vi "svx_Polar_Property_Dialog.vi"(0 "Data in":T1, 1 "Container State in":T2 caption="Container State", 2 "Polar Plot":refnum<vi>, 3 "Plot Legend":refnum<vi>, 4 "z scale graph ref in":refnum<vi>, 5 "This VI":refnum<vi>, 6 "State in":T4={"Property Name"=[], "Container bounds"={"Width"=550, "Height"=250}, "Scale range"={"Maximum"=1.0, "Increment"=1.0}, "PointIdx"=0, "Marker list"=[], "Color settings"={"Arrow color"=16860, "Magnitude major grid"=13816530, "Magnitude minor grid"=16777216, "Phase grid"=13816530, "Phase scale marker text"=0}, "Magnitude scale name"="Magnitude", "Magnitude scale format string"="%#.2e", "MagnitudeScale:Visible"=TRUE, "MagnitudeScaleLabel:Visible"=TRUE, "PhaseScale:Visible"=TRUE, "Marker:Visible"=TRUE, "Cursor:Visible"=FALSE, "CursorName:Visible"=TRUE, "Autoscale"=TRUE, "Marker color"=16860, "Line color"=16711680, "Cursor color"=16711680, "Magnitude scale marker color"=0, "Plot.Line Style"=0, "Plot.Line Width"=0, "Plot.Point Style"=0, "Cursor.Line Style"=0, "Cursor.Line Width"=0, "Cursor.Point Style"=0, "Cursor.Style"=4, "Marker.Point Style"=2, "Point/fill color"=16711680, "Background color"=16777225, "Cursor name"="", "Cursor Release"=refnum, "Scale Range Change"=refnum, "data size(s)"=[], "Selectors:Visible"=TRUE, "Selector:ring Strings"={"Selector:Custom Strings"=FALSE, "Selector:Row Strings []"=[], "Selector:Column Strings []"=[], "User:Row Strings []"=[], "User:Column Strings []"=[]}, "Lock Cursor Info Position"=FALSE, "CursLoc"={"magnitude"=0.0, "phase"=0.0, "time/rev/RPM"=0.0}, "Plot Area:Position"={"Left"=0, "Top"=0}, "Plot Area:Size"={"Width"=0, "Height"=0}, "Marker.Style"=0, "Indication Arcs"=[], "Arc.Selector"=0, "customized marker"=[], "tree Width"=0, " Parents Tags"=[], "Children Tags"=[], "open?"=[], "index"=[{"row index"=0, "column index"=0}], "Label"="", "custom strings changed"=FALSE, "Owning VI"=refnum, "Legend BG color"=16777225, "Legend font color"=0, "column Width"=203, "attribute"=variant} caption="State", 7 "Action in":T3, 8 "acceptance region only?":bool, 9 "Cursor Info":refnum<vi>) -> (12 "State out":T4={"Property Name"=[], "Container bounds"={"Width"=550, "Height"=250}, "Scale range"={"Maximum"=1.0, "Increment"=1.0}, "PointIdx"=0, "Marker list"=[], "Color settings"={"Arrow color"=16860, "Magnitude major grid"=13816530, "Magnitude minor grid"=16777216, "Phase grid"=13816530, "Phase scale marker text"=0}, "Magnitude scale name"="Magnitude", "Magnitude scale format string"="%#.2e", "MagnitudeScale:Visible"=TRUE, "MagnitudeScaleLabel:Visible"=TRUE, "PhaseScale:Visible"=TRUE, "Marker:Visible"=TRUE, "Cursor:Visible"=FALSE, "CursorName:Visible"=TRUE, "Autoscale"=TRUE, "Marker color"=16860, "Line color"=16711680, "Cursor color"=16711680, "Magnitude scale marker color"=0, "Plot.Line Style"=0, "Plot.Line Width"=0, "Plot.Point Style"=0, "Cursor.Line Style"=0, "Cursor.Line Width"=0, "Cursor.Point Style"=0, "Cursor.Style"=4, "Marker.Point Style"=2, "Point/fill color"=16711680, "Background color"=16777225, "Cursor name"="", "Cursor Release"=refnum, "Scale Range Change"=refnum, "data size(s)"=[], "Selectors:Visible"=TRUE, "Selector:ring Strings"={"Selector:Custom Strings"=FALSE, "Selector:Row Strings []"=[], "Selector:Column Strings []"=[], "User:Row Strings []"=[], "User:Column Strings []"=[]}, "Lock Cursor Info Position"=FALSE, "CursLoc"={"magnitude"=0.0, "phase"=0.0, "time/rev/RPM"=0.0}, "Plot Area:Position"={"Left"=0, "Top"=0}, "Plot Area:Size"={"Width"=0, "Height"=0}, "Marker.Style"=0, "Indication Arcs"=[], "Arc.Selector"=0, "customized marker"=[], "tree Width"=0, " Parents Tags"=[], "Children Tags"=[], "open?"=[], "index"=[{"row index"=0, "column index"=0}], "Label"="", "custom strings changed"=FALSE, "Owning VI"=refnum, "Legend BG color"=16777225, "Legend font color"=0, "column Width"=203, "attribute"=variant} caption="State", 13 "Action out":T3, 14 "Data out":T1)   [LabVIEW 2017, in "SVX Polar Plot.xctl"]
uses:
  <vilib>/addons/_XControls/Polar Plot/SVX Polar Plot.xctl
  <vilib>/addons/_XControls/Polar Plot/subVIs/svx_Polar_Plot_Internal_State.ctl
  <vilib>/addons/_XControls/Polar Plot/subVIs/svx_Polar_Indication_Arcs.ctl
  <vilib>/addons/_XControls/Polar Plot/subVIs/svx_Polar_Customized_Markers.ctl
  <vilib>/_xctls/Action.ctl
  <vilib>/_xctls/Container State.ctl
  <vilib>/addons/_XControls/Polar Plot/subVIs/svx_Polar_Plot_Data.ctl
  <vilib>/addons/_XControls/Polar Plot/subVIs/svx_Polar_Exe_Tasks.ctl
  <vilib>/_xctls/XControlSupport.lvlib
panel:
  out "update maximum value":bool
  in  "Help":bool
  in  "Cancel":bool
  in  "OK":bool
  in  "Main Tab":T7(tab)
  in  "Plot Legend Font.Color":u32(colorbox)=16777222 caption="Legend font"
  in  "Plot Legend Background.Color":u32(colorbox)=16777225 caption="Legend background"
  in  "Background.Color":u32(colorbox)=16777225 caption="Background"
  in  "Enable State":T8(radio)
  in  "Arrow.Color":u32(colorbox)=16860 caption="Arrow color"
  in  "Label.Visible":bool=TRUE
  in  "Label.Text":string="Polar Plot"
  in  "Caption.Visible":bool
  in  "Caption.Text":string="Polar Plot"
  in  "Hide trailing zeros":bool=TRUE
  in  "Digits":u8=2
  in  "Precision Type":u16(ring) items=["Digits of precision", "Significant digits"]
  in  "Type":i32(listbox)=2
  in  "Point/Fill.Color":u32(colorbox)=16860 caption="Point/Fill"
  in  "Marker.Point Style":T9 caption="Point Style"
  in  "Line.Color":u32(colorbox)=16860 caption="Line color"
  in  "Plot.Point Style":T9 caption="Point Style"
  in  "Plot.Line Style":T10 caption="Line Style"
  in  "Plot.Line Width":T11 caption="Line Width"
  in  "Marker.Color":u32(colorbox)=16711680 caption="Marker color"
  in  "Marker.Visible":bool=TRUE caption="Show scale label"
  in  "Marker.Style":T12 caption="Cursor Style"
  in  "Magnitude Minor Grid.Color":u32(colorbox)=16777216 caption="Magnitude minor grid"
  in  "Phase Scale.Visible":bool=TRUE caption="Show scale"
  in  "Magnitude Scale Marker Text.Color":u32(colorbox) caption="Magnitude scale marker text"
  in  "Phase Grid.Color":u32(colorbox)=13816530 caption="Phase grid"
  in  "Magnitude Major Grid.Color":u32(colorbox)=13816530 caption="Magnitude major grid"
  in  "Phase Scale Marker Text.Color":u32(colorbox) caption="Phase scale marker text"
  in  "Magnitude Scale Label.Visible":bool=TRUE caption="Show scale label"
  in  "Magnitude Range:Maximum":dbl=10.0 caption="Maximum" min=0.0 format="%0.2f"
  in  "Magnitude.Scale Fit":bool caption="Autoscale"
  in  "Magnitude Scale.Visible":bool=TRUE caption="Show scale"
  in  "Magnitude.Text":string caption="Name"
  in  "Cursor Info Position.Lock":bool caption="Show scale label"
  in  "Cursor.Visible":bool=TRUE caption="Show scale label"
  in  "Cursor.Color":u32(colorbox)=16711680 caption="Cursor color"
  in  "Cursor Info.Visible":bool=TRUE caption="Show scale label"
  in  "Cursor.Style":T12 caption="Cursor Style"
  in  "Cursor.Line Width":T11 caption="Line Width"
  in  "Cursor.Line Style":T10 caption="Line Style"
  in  "Cursor.Point Style":T9 caption="Point Style"
  in  "AR.Selector":u16(ring) caption="Indication Arc" items=["Acceptance Region 0"]
  in  "AR.Fill Color":u32(colorbox)=16777216 caption="Fill color"
  in  "AR.Name":string caption="Name"
  in  "AR.Remove":bool
  in  "AR.Add":bool
  in  "AR.Style":T10 caption="Line Style"
  in  "AR.Width":T11 caption="Line Width"
  in  "AR.Start Radius":dbl caption="Start radius"
  in  "AR.Color":u32(colorbox)=16711680 caption="Border color"
  in  "AR.Start Angle":i16 caption="Start angle" min=-360 max=360
  in  "AR.End Angle":i16=360 caption="End angle" min=-360 max=360
  in  "AR.Visible":bool
  in  "AR.End Radius":dbl caption="End radius"
  in  "Tip strip":string
  in  "Description":string
  # "Label"
  # "Caption"
  # "Enabled State"
  # "Color Scheme"
  # "Magnitude"
  # "Plot"
  # "Color"
  # "Marker"
  # "Magnitude"
  # "Phase"
  # "Cursor"
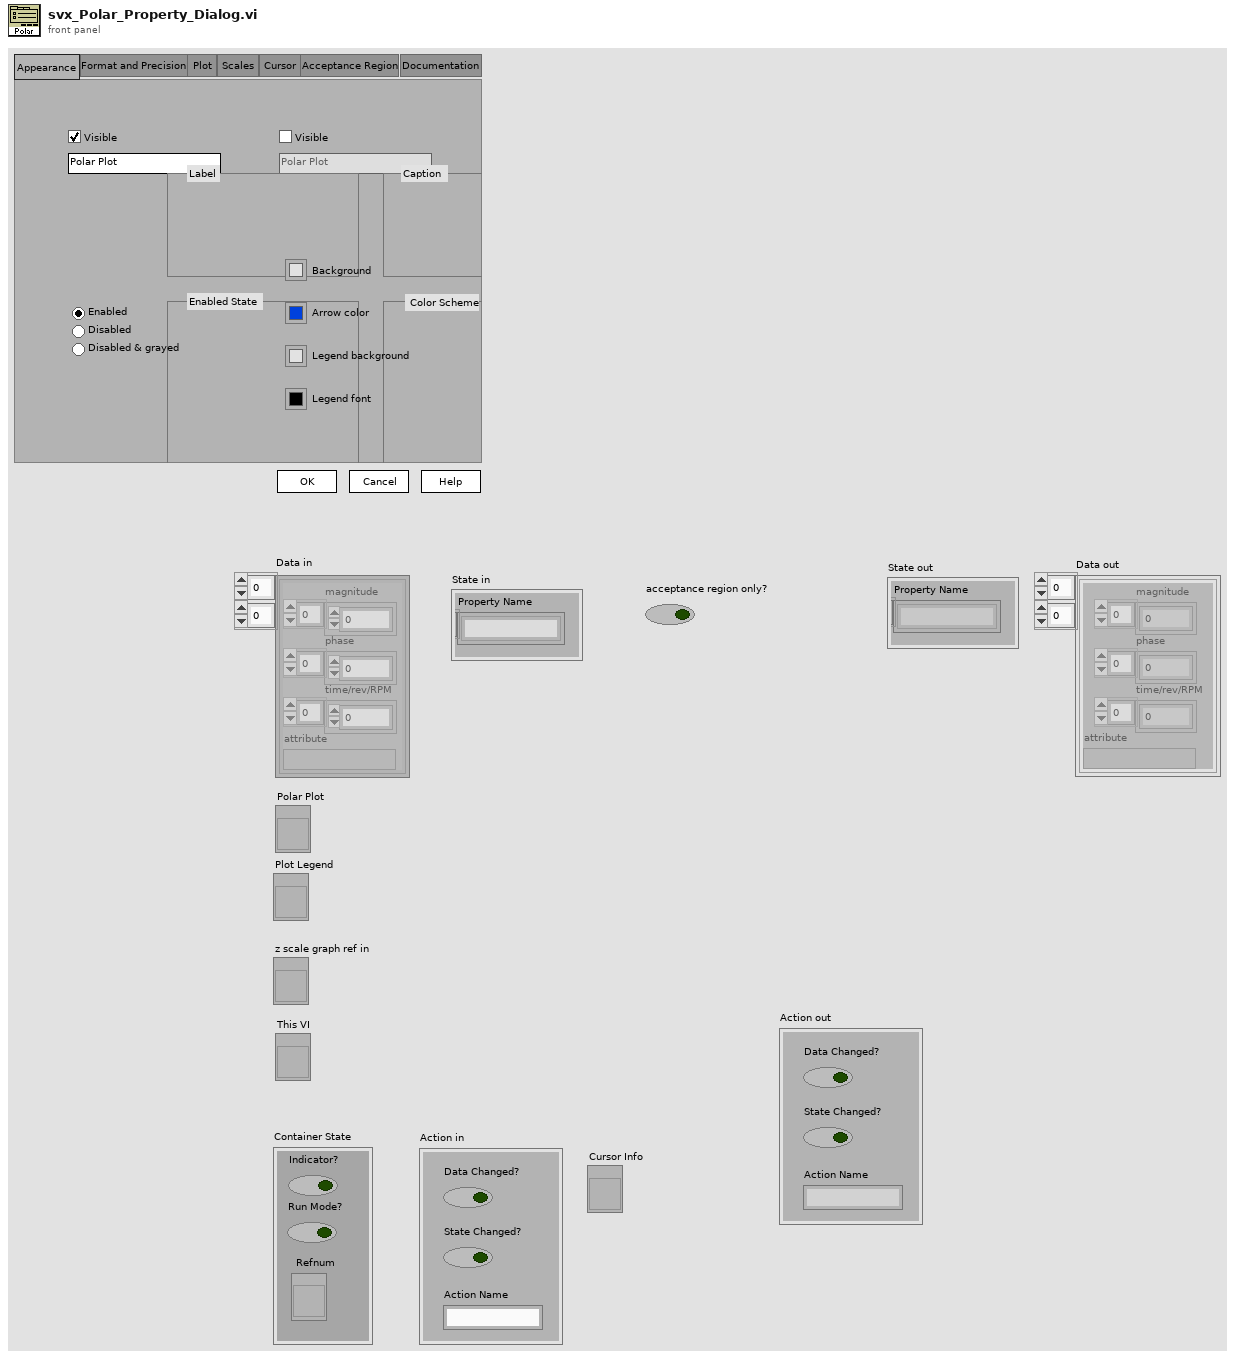
[diagram p1: front panel]
types:
  T1 = typedef "SVX Polar Plot.xctl/svx_Polar_Plot_Data.ctl" = cluster{"magnitude":dbl[], "phase":dbl[], "time/rev/RPM":dbl[], "attribute":variant}[][]
  T2 = typedef "XControlSupport.lvlib/Container State.ctl" = cluster{"Indicator?":bool, "Run Mode?":bool, " Refnum":refnum<vi>}
  T3 = typedef "XControlSupport.lvlib/Action.ctl" = cluster{"Data Changed?":bool, "State Changed?":bool, "Action Name":string}
  T4 = typedef "SVX Polar Plot.xctl/svx_Polar_Plot_Internal_State.ctl" = cluster{"Property Name":string[], "Container bounds":cluster{"Width":u32, "Height":u32}, "Scale range":cluster{"Maximum":dbl, "Increment":dbl}, "PointIdx":i32, "Marker list":cluster{"Name":string, "Color":u32, "Style":u8, "Point Style":u8, "Name Visible":bool, "Allow Drag":bool, "Annotation Mode":u32, "Plot":i32, "Index":i32, "Position":cluster{"X":dbl, "Y":dbl}, "X Scale":u32, "Y Scale":u32, "Show Arrow":bool, "Lock Name":bool, "Plot Area":i32, "Label Offset":cluster{"X":dbl, "Y":dbl}}[], "Color settings":cluster{"Arrow color":u32, "Magnitude major grid":u32, "Magnitude minor grid":u32, "Phase grid":u32, "Phase scale marker text":u32}, "Magnitude scale name":string, "Magnitude scale format string":string, "MagnitudeScale:Visible":bool, "MagnitudeScaleLabel:Visible":bool, "PhaseScale:Visible":bool, "Marker:Visible":bool, "Cursor:Visible":bool, "CursorName:Visible":bool, "Autoscale":bool, "Marker color":u32, "Line color":u32, "Cursor color":u32, "Magnitude scale marker color":u32, "Plot.Line Style":i32, "Plot.Line Width":i32, "Plot.Point Style":i32, "Cursor.Line Style":i32, "Cursor.Line Width":i32, "Cursor.Point Style":i32, "Cursor.Style":i32, "Marker.Point Style":i32, "Point/fill color":u32, "Background color":u32, "Cursor name":string, "Cursor Release":refnum<user-event>, "Scale Range Change":refnum<user-event>, "data size(s)":i32[], "Selectors:Visible":bool, "Selector:ring Strings":cluster{"Selector:Custom Strings":bool, "Selector:Row Strings []":string[], "Selector:Column Strings []":string[], "User:Row Strings []":string[], "User:Column Strings []":string[]}, "Lock Cursor Info Position":bool, "CursLoc":cluster{"magnitude":dbl, "phase":dbl, "time/rev/RPM":dbl}, "Plot Area:Position":cluster{"Left":i32, "Top":i32}, "Plot Area:Size":cluster{"Width":u32, "Height":u32}, "Marker.Style":i32, "Indication Arcs":T5, "Arc.Selector":u16, "customized marker":T6, "tree Width":u32, " Parents Tags":string[], "Children Tags":string[], "open?":bool[], "index":cluster{"row index":i32, "column index":i32}[], "Label":string, "custom strings changed":bool, "Owning VI":refnum<vi>, "Legend BG color":u32, "Legend font color":u32, "column Width":u32, "attribute":variant}
  T5 = typedef "SVX Polar Plot.xctl/svx_Polar_Indication_Arcs.ctl" = cluster{"Name":string, "Start radius":dbl, "End radius":dbl, "Line Style":i32, "Line Width":i32, "Border color":u32, "Fill color":u32, "Start angle":i16, "End angle":i16, "Visible":bool}[]
  T6 = typedef "SVX Polar Plot.xctl/svx_Polar_Customized_Markers.ctl" = cluster{"Name":string, "Color":u32, "Style":u8, "Point Style":u8, "Name Visible":bool, "Allow Drag":bool, "Annotation Mode":u32, "Plot":i32, "Index":i32, "Position":cluster{"Magnitude":dbl, "Phase":dbl}, "X Scale":u32, "Y Scale":u32, "Show Arrow":bool, "Lock Name":bool, "Plot Area":i32, "Label Offset":cluster{"Magnitude":dbl, "Phase":dbl}}[]
  T7 = enum32{"Appearance", "Format and Precision", "Plot", "Scales", "Cursor", "Acceptance Region", "Documentation"}
  T8 = enum32{"Enabled", "Disabled", "Disabled & grayed"}
  T9 = cluster{"OK Button 17":bool, "OK Button":bool, "OK Button 2":bool, "OK Button 3":bool, "OK Button 4":bool, "OK Button 5":bool, "OK Button 6":bool, "OK Button 7":bool, "OK Button 8":bool, "OK Button 9":bool, "OK Button 10":bool, "OK Button 11":bool, "OK Button 12":bool, "OK Button 13":bool, "OK Button 14":bool, "OK Button 15":bool, "OK Button 16":bool}
  T10 = cluster{"OK Button":bool, "OK Button 2":bool, "OK Button 3":bool, "OK Button 4":bool, "OK Button 5":bool}
  T11 = cluster{"OK Button 2":bool, "OK Button 3":bool, "OK Button 4":bool, "OK Button 5":bool, "OK Button 6":bool, "OK Button 7":bool}
  T12 = cluster{"OK Button 17":bool, "OK Button":bool, "OK Button 2":bool, "OK Button 5":bool, "OK Button 13":bool, "OK Button 10":bool, "OK Button 6":bool, "OK Button 9":bool, "OK Button 14":bool}
  T13 = cluster{"Label.Text":string, "Caption.Text":string, "Label.Visible":bool, "Caption.Visible":bool, "Disabled":u8, "Desc":string, "TipStrip":string}
  T14 = cluster{"Name":string, "Start radius":dbl, "End radius":dbl, "Line Style":i32, "Line Width":i32, "Border color":u32, "Fill color":u32, "Start angle":i16, "End angle":i16, "Visible":bool}
  T15 = typedef "SVX Polar Plot.xctl/svx_Polar_Exe_Tasks.ctl" = enum16{"[Data] Update Data", "[Scale] Update Polar Scale", "[Scale] Autoscale", "[Legend] Update Legend", "[Cursor] Cursor Release", "[Pane] Change Minimum Size", "[Annt] Upodate Annotation", "[Plot] Appearance", "[Cursor] Visibility", "[Cursor] Appearance", "[Cursor] Index", "[Scale] MagnitudeVisibility", "[Scale] PhaseVisibility", "[Scale] PhaseAppearance", "[Scale] MagnitudeApperance", "[Plot] AcceptanceRegion", "[Scale] RangeChange", "[Marker] Appearance", "[Marker] List", "[Marker] Visibility", "[Legend] Visibility", "[Legend] Color", "[Data] Index", "[Legend] Update String", "[Cursor] Trigger Event", "[Scale] Trigger Event", "[Data] Clear Graph"}
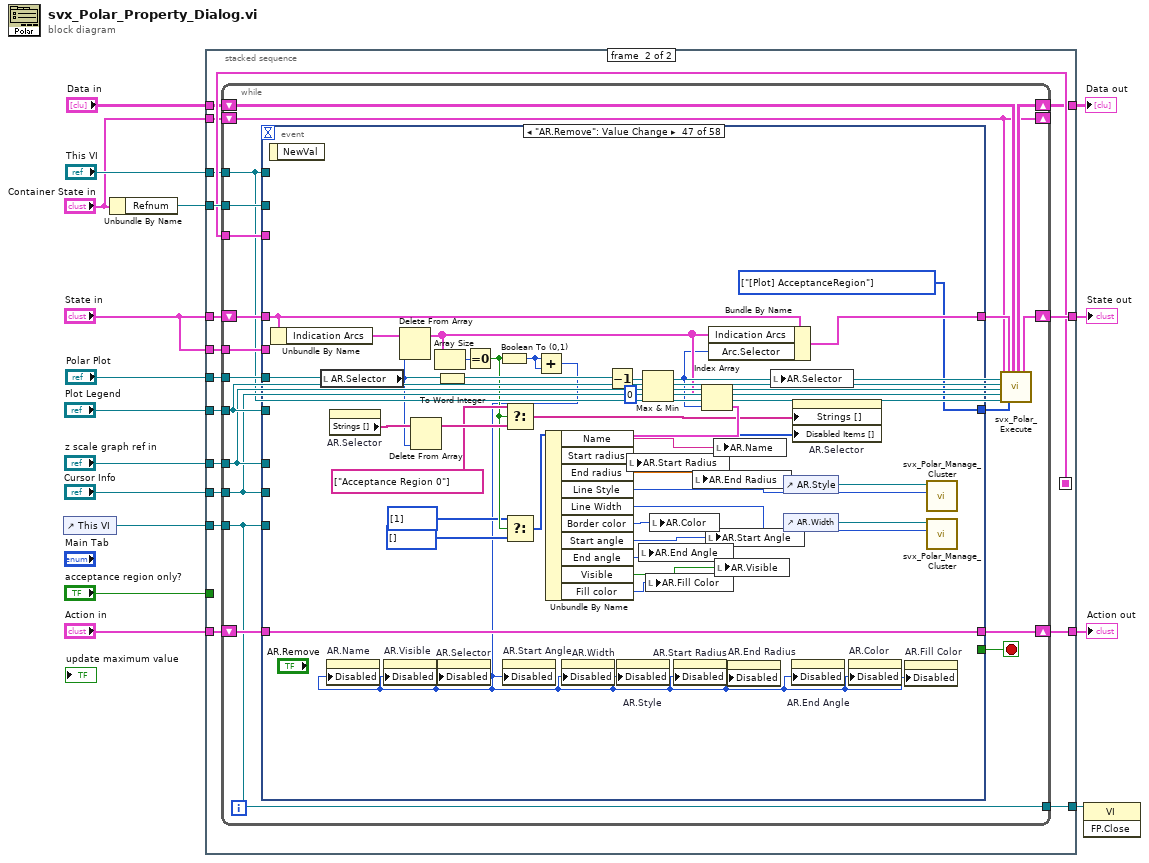
[diagram p0: block diagram]
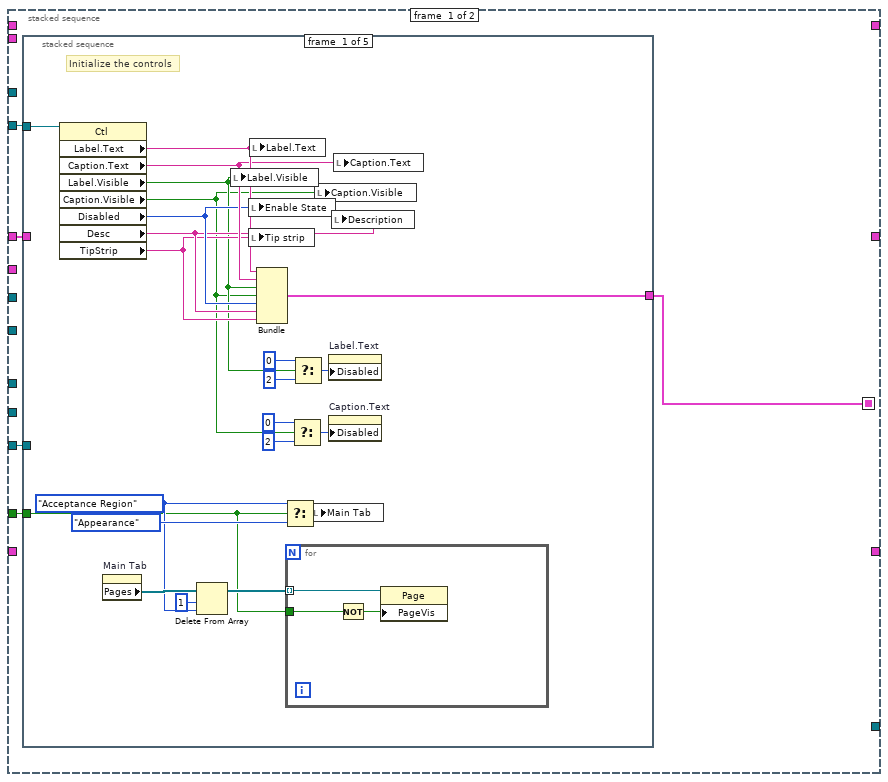
[diagram p2: hidden frame]
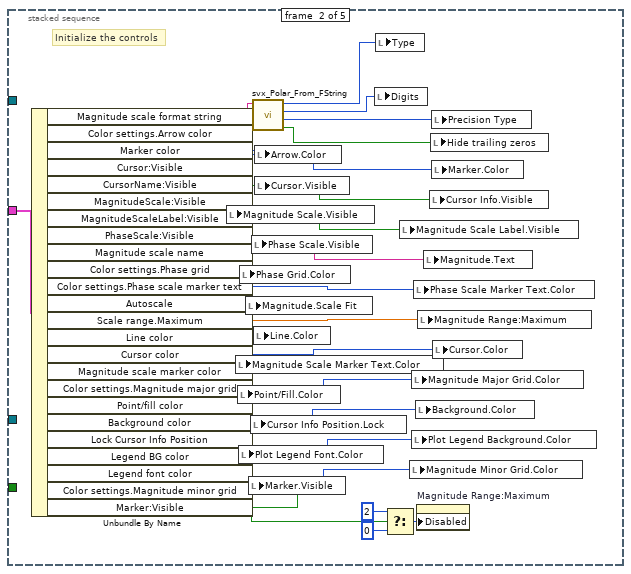
[diagram p3: hidden frame]
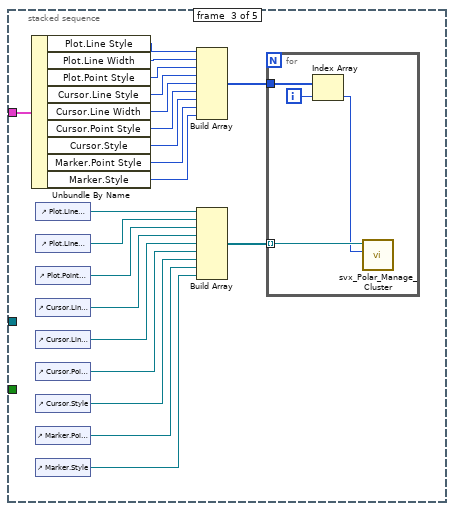
[diagram p4: hidden frame]
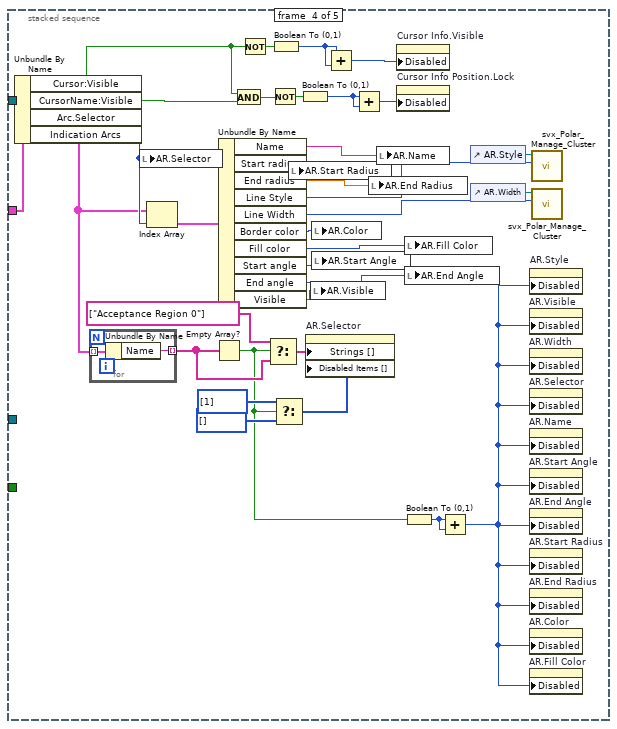
[diagram p5: hidden frame]
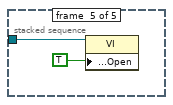
[diagram p6: hidden frame]
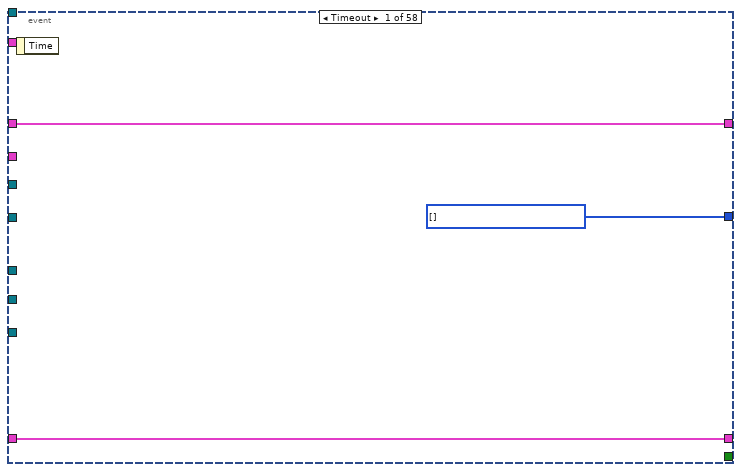
[diagram p7: hidden frame]
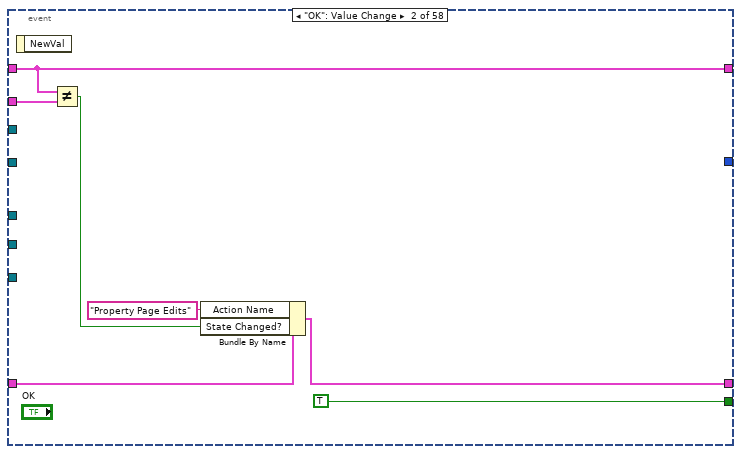
[diagram p8: hidden frame]
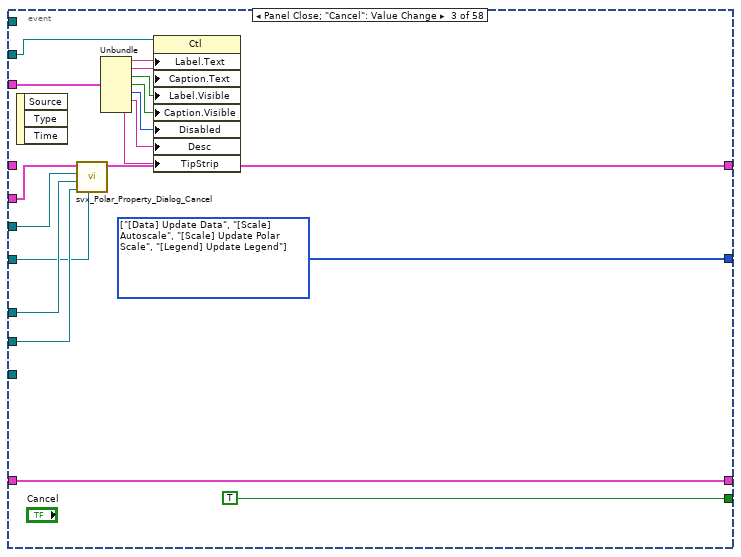
[diagram p9: hidden frame]
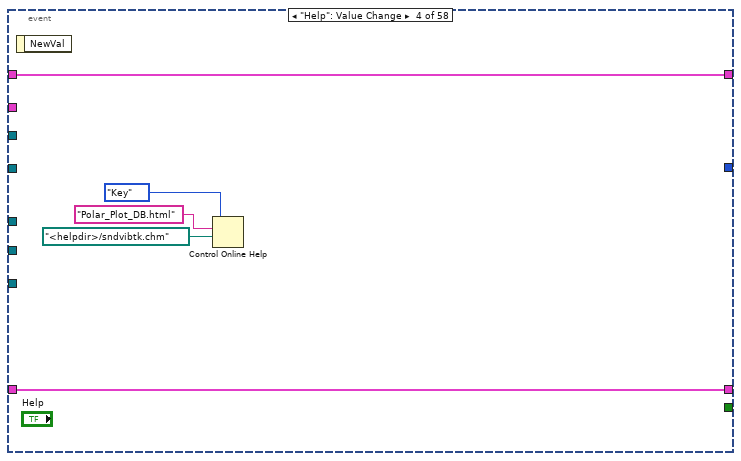
[diagram p10: hidden frame]
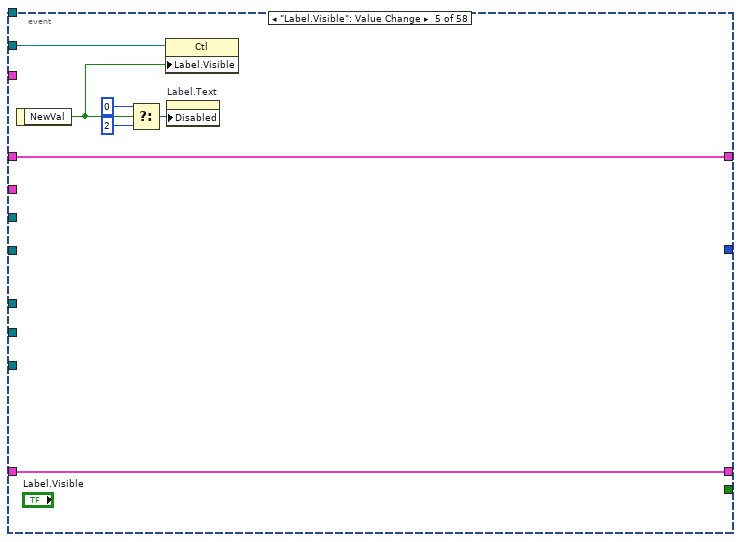
[diagram p11: hidden frame]
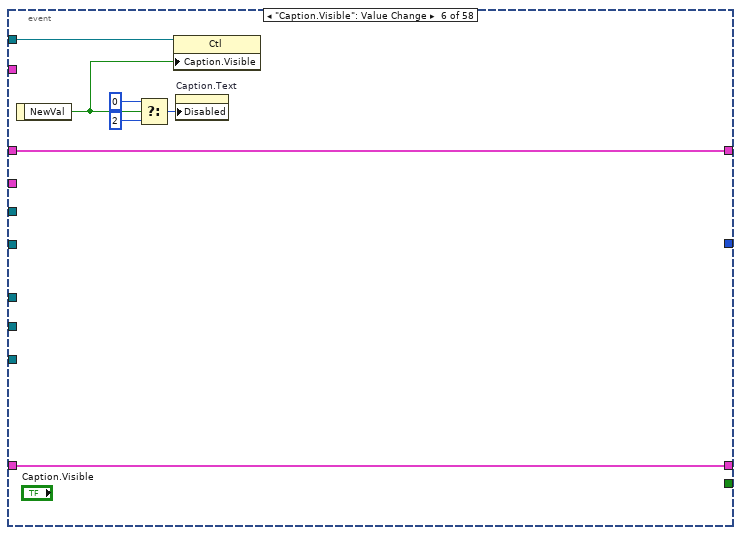
[diagram p12: hidden frame]
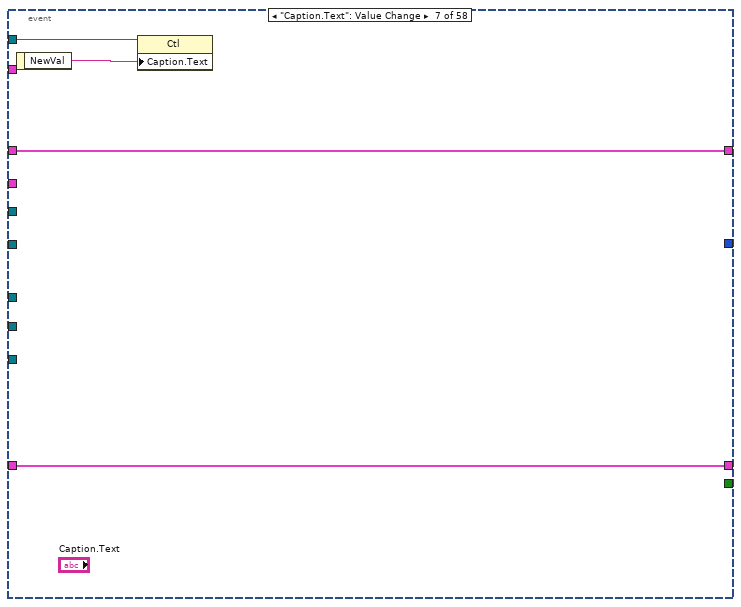
[diagram p13: hidden frame]
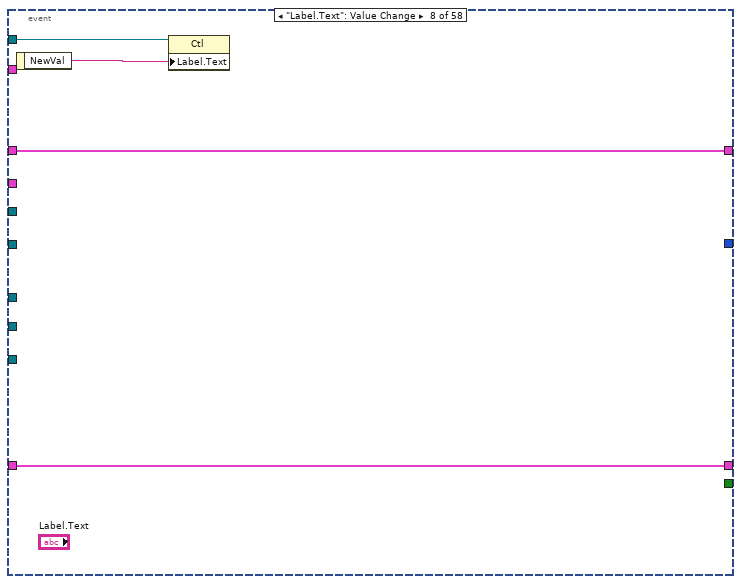
[diagram p14: hidden frame]
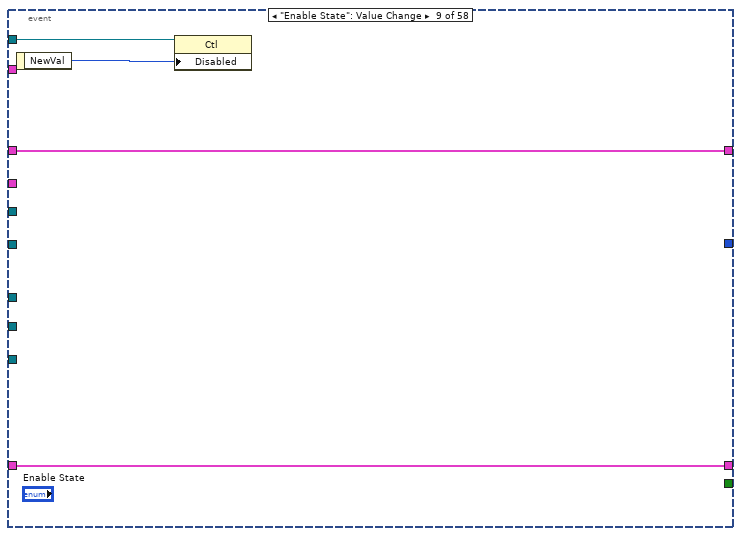
[diagram p15: hidden frame]
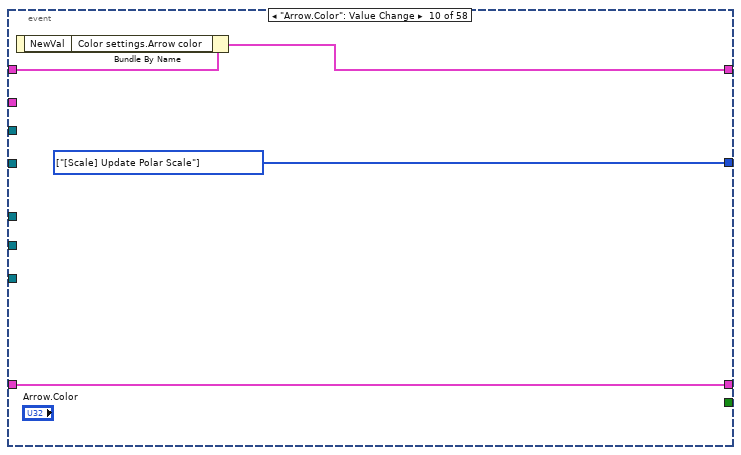
[diagram p16: hidden frame]
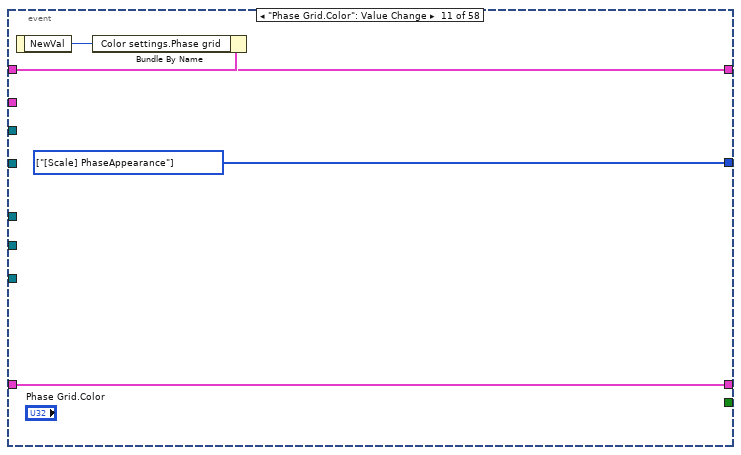
[diagram p17: hidden frame]
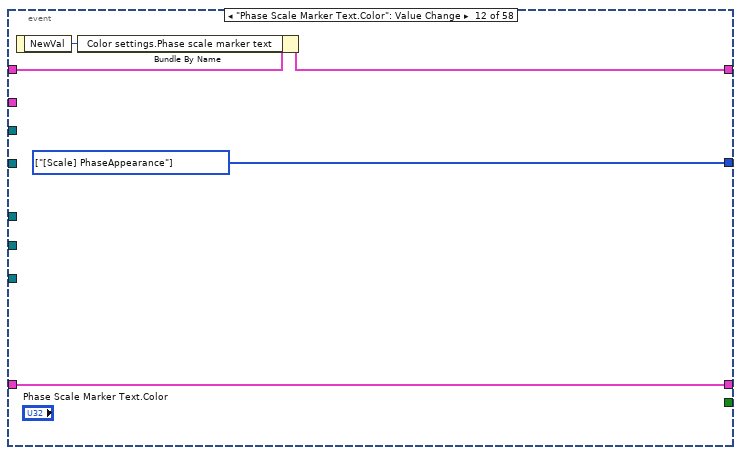
[diagram p18: hidden frame]
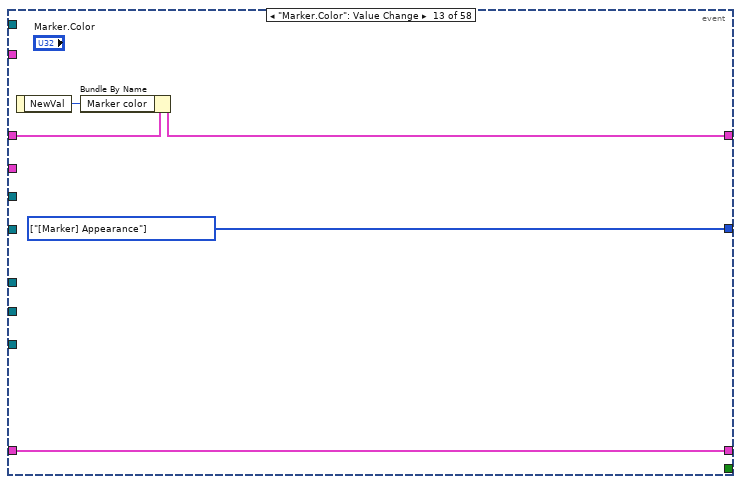
[diagram p19: hidden frame]
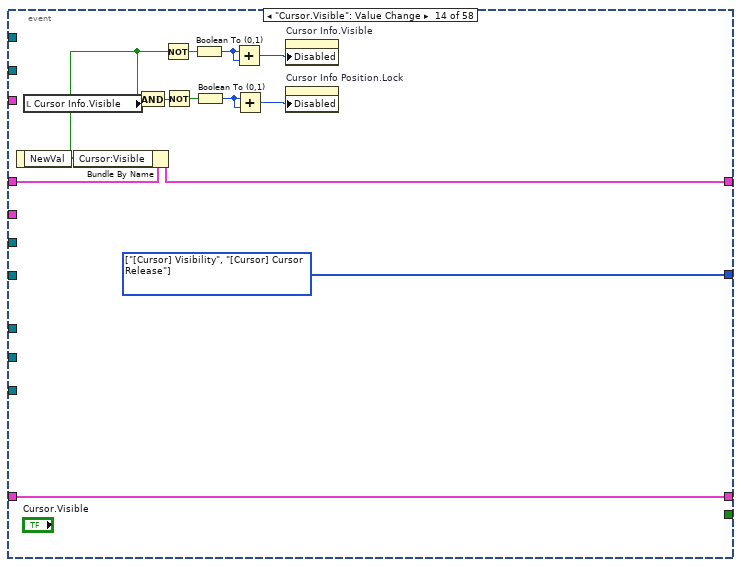
[diagram p20: hidden frame]
diagram:
  n1 = control-ref of="This VI"() -> (w7:refnum<vi>)
  n2 = Unbundle By Name("Container State in") -> ("Refnum"=w15:refnum<vi>)
  n3 = stacked-sequence {
    seq-local: [w19 _] -> [_ w150]
    tunnel: "State in" -> [w21 w158]
    tunnel: [_ w157] -> w16
    tunnel: w15 -> [w20 w156]
    tunnel: "Action in" -> [_ w155]
    tunnel: [_ w154] -> w13
    tunnel: "Polar Plot" -> [_ w153]
    tunnel: "z scale graph ref in" -> [_ w152]
    tunnel: "State in" -> [_ w151]
    tunnel: "Cursor Info" -> [_ w149]
    tunnel: "Plot Legend" -> [_ w148]
    tunnel: "acceptance region only?" -> [w18 _]
    tunnel: w7 -> [w17 w147]
    tunnel: [_ w146] -> w6
    tunnel: "This VI" -> [_ w145]
    tunnel: "Data in" -> [_ w144]
    tunnel: [_ w143] -> w3
    tunnel: "Container State in" -> [_ w142]
    frame #0 {
      n4 = stacked-sequence {
        tunnel: w20 -> [w43 _ _ _ _]
        tunnel: w21 -> [_ w78 w99 w137 _]
        tunnel: [w37 _ _ _ _] -> w19
        tunnel: w18 -> [w30 _ _ _ _]
        tunnel: w17 -> [_ _ _ _ w141]
        frame #0 {
          w32 = T7."Acceptance Region" ("Main Tab")
          # "Initialize the controls"
          n5 = property class="Ctl"(reference=w43) -> ("Label.Text"=w42:string, "Caption.Text"=w41:string, "Label.Visible"=w26:bool, "Caption.Visible"=w22:bool, "Disabled"=w40:u8, "Desc"=w39:string, "TipStrip"=w38:string)  [unwired: 1 in, 2 out]
          n6 = property on="Main Tab" class="TabCtl (strict)"() -> ("Pages"=w34:refnum<vi>[])  [unwired: 2 in, 2 out]
          n7 = Delete From Array(array=w34, length=1, index=w32) -> (array with subset deleted=w31:refnum<vi>[])  [unwired: 1 out]
          n8 = local write "Label.Visible"(w26) -> ()
          n9 = local write "Enable State"(w40) -> ()
          n10 = local write "Tip strip"(w38) -> ()
          n11 = local write "Label.Text"(w42) -> ()
          n12 = Bundle("Label.Text"=w42, "Caption.Text"=w41, "Label.Visible"=w26, "Caption.Visible"=w22, "Disabled"=w40, "Desc"=w39, "TipStrip"=w38) -> (w37:T13)  [unwired: 1 in]
          n13 = Select(t=w32, s=w30, f=T7."Appearance" ("Main Tab")) -> (s? t:f=w35:T7)
          n14 = for {
            tunnel: w31 -> [w46] mode=indexing
            tunnel: w30 -> [w44]
            n15 = Not(x=w44) -> (.not. x?=w45:bool)
            n16 = property class="Page"(reference=w46, "PageVis"=w45) -> ()  [unwired: 1 in, 2 out]
          }
          n17 = Select(t=u8 0 ("Disabled"), s=w22, f=u8 2 ("Disabled")) -> (s? t:f=w23:u8)
          n18 = Select(t=u8 0 ("Disabled"), s=w26, f=u8 2 ("Disabled")) -> (s? t:f=w27:u8)
          n19 = local write "Main Tab"(w35) -> ()
          n20 = local write "Caption.Visible"(w22) -> ()
          n21 = property on="Label.Text" class="Str"("Disabled"=w27) -> ()  [unwired: 2 in, 2 out]
          n22 = property on="Caption.Text" class="Str"("Disabled"=w23) -> ()  [unwired: 2 in, 2 out]
          n23 = local write "Description"(w39) -> ()
          n24 = local write "Caption.Text"(w41) -> ()
        }
        frame #1 {
          # "Initialize the controls"
          n25 = Unbundle By Name(w78) -> ("Magnitude scale format string"=w66:string, "Color settings.Arrow color"=w77:u32, "Marker color"=w76:u32, "Cursor:Visible"=w75:bool, "CursorName:Visible"=w74:bool, "MagnitudeScale:Visible"=w73:bool, "MagnitudeScaleLabel:Visible"=w72:bool, "PhaseScale:Visible"=w71:bool, "Magnitude scale name"=w70:string, "Color settings.Phase grid"=w69:u32, "Color settings.Phase scale marker text"=w68:u32, "Autoscale"=w52:bool, "Scale range.Maximum"=w67:dbl, "Line color"=w61:u32, "Cursor color"=w60:u32, "Magnitude scale marker color"=w59:u32, "Color settings.Magnitude major grid"=w58:u32, "Point/fill color"=w57:u32, "Background color"=w56:u32, "Lock Cursor Info Position"=w55:bool, "Legend BG color"=w50:u32, "Legend font color"=w49:u32, "Color settings.Magnitude minor grid"=w48:u32, "Marker:Visible"=w47:bool)
          n26 = local write "Magnitude Scale.Visible"(w73) -> ()
          n27 = local write "Magnitude Scale Marker Text.Color"(w59) -> ()
          n28 = local write "Point/Fill.Color"(w57) -> ()
          n29 = local write "Plot Legend Font.Color"(w49) -> ()
          n30 = local write "Phase Grid.Color"(w69) -> ()
          n31 = local write "Magnitude.Scale Fit"(w52) -> ()
          n32 = local write "Marker.Visible"(w47) -> ()
          n33 = local write "Cursor Info Position.Lock"(w55) -> ()
          n34 = local write "Phase Scale.Visible"(w71) -> ()
          n35 = call <vilib>:"svx_Polar_From_FString.vi"("Format string"=w66) -> ("trailing zeros"=w62:bool, "Precision Type"=w63:u16, "Digits"=w64:u8, "Type"=w65:i32)  [unwired: 7 in]
          n36 = local write "Line.Color"(w61) -> ()
          n37 = local write "Arrow.Color"(w77) -> ()
          n38 = local write "Cursor.Visible"(w75) -> ()
          n39 = local write "Digits"(w64) -> ()
          n40 = local write "Type"(w65) -> ()
          n41 = Select(t=u8 2 ("Disabled"), s=w52, f=u8 0 ("Disabled")) -> (s? t:f=w51:u8)
          n42 = local write "Magnitude Scale Label.Visible"(w72) -> ()
          n43 = local write "Magnitude Minor Grid.Color"(w48) -> ()
          n44 = local write "Magnitude Major Grid.Color"(w58) -> ()
          n45 = local write "Plot Legend Background.Color"(w50) -> ()
          n46 = local write "Phase Scale Marker Text.Color"(w68) -> ()
          n47 = local write "Background.Color"(w56) -> ()
          n48 = property on="Magnitude Range:Maximum" class="DigNum (strict)"("Disabled"=w51) -> ()  [unwired: 2 in, 2 out]
          n49 = local write "Magnitude Range:Maximum"(w67) -> ()
          n50 = local write "Magnitude.Text"(w70) -> ()
          n51 = local write "Cursor Info.Visible"(w74) -> ()
          n52 = local write "Hide trailing zeros"(w62) -> ()
          n53 = local write "Precision Type"(w63) -> ()
          n54 = local write "Marker.Color"(w76) -> ()
          n55 = local write "Cursor.Color"(w60) -> ()
        }
        frame #2 {
          n56 = Unbundle By Name(w99) -> ("Plot.Line Style"=w98:i32, "Plot.Line Width"=w97:i32, "Plot.Point Style"=w96:i32, "Cursor.Line Style"=w95:i32, "Cursor.Line Width"=w94:i32, "Cursor.Point Style"=w93:i32, "Cursor.Style"=w92:i32, "Marker.Point Style"=w91:i32, "Marker.Style"=w90:i32)
          n57 = control-ref of="Plot.Line Style"() -> (w89:refnum<vi>)
          n58 = control-ref of="Plot.Line Width"() -> (w88:refnum<vi>)
          n59 = control-ref of="Plot.Point Style"() -> (w87:refnum<vi>)
          n60 = control-ref of="Cursor.Line Style"() -> (w86:refnum<vi>)
          n61 = control-ref of="Cursor.Line Width"() -> (w85:refnum<vi>)
          n62 = control-ref of="Cursor.Point Style"() -> (w84:refnum<vi>)
          n63 = control-ref of="Cursor.Style"() -> (w83:refnum<vi>)
          n64 = control-ref of="Marker.Point Style"() -> (w82:refnum<vi>)
          n65 = control-ref of="Marker.Style"() -> (w81:refnum<vi>)
          n66 = Build Array(w98, w97, w96, w95, w94, w93, w92, w91, w90) -> (w80:i32[])
          n67 = Build Array(w89, w88, w87, w86, w85, w84, w83, w82, w81) -> (w79:refnum<vi>[])
          n68 = for {
            tunnel: w80 -> [w102]
            tunnel: w79 -> [w103] mode=indexing
            i -> [w101]
            n69 = Index Array(array=w102, index=w101) -> (element=w100:i32)
            n70 = call <vilib>:"svx_Polar_Manage_Cluster.vi"("index"=w100, "Clust Refnum"=w103) -> ()  [unwired: 10 in]
          }
        }
        frame #3 {
          n71 = Unbundle By Name(w137) -> ("Cursor:Visible"=w130:bool, "CursorName:Visible"=w129:bool, "Arc.Selector"=w117:u16, "Indication Arcs"=w115:T5)
          n72 = for {
            tunnel: w115 -> [w139] mode=indexing
            tunnel: [w138] -> w114 mode=indexing
            n73 = Unbundle By Name(w139) -> ("Name"=w138:string)
          }
          n74 = local write "AR.Selector"(w117) -> ()
          n75 = Index Array(array=w115, index=w117) -> (element=w116:T14)
          n76 = Empty Array?(array=w114) -> (empty?=w107:bool)
          n77 = Unbundle By Name(w116) -> ("Name"=w127:string, "Start radius"=w126:dbl, "End radius"=w106:dbl, "Line Style"=w120:i32, "Line Width"=w119:i32, "Border color"=w125:u32, "Fill color"=w104:u32, "Start angle"=w124:i16, "End angle"=w123:i16, "Visible"=w122:bool)
          n78 = And(x=w130, y=w129) -> (x .and. y?=w128:bool)
          n79 = Not(x=w130) -> (.not. x?=w133:bool)
          n80 = Select(t=string[] ["Acceptance Region 0"], s=w107, f=w114) -> (s? t:f=w112:string[])
          n81 = Not(x=w128) -> (.not. x?=w132:bool)
          n82 = Boolean To (0,1)(Boolean=w133) -> (0, 1=w134:i16)
          n83 = Select(t=i32[] [1] ("Disabled Items []"), s=w107, f=i32[] [] ("Disabled Items []")) -> (s? t:f=w109:i32[])
          n84 = local write "AR.Start Radius"(w126) -> ()
          n85 = Boolean To (0,1)(Boolean=w132) -> (0, 1=w136:i16)
          n86 = property on="AR.Selector" class="Ring (strict)"("Strings []"=w112, "Disabled Items []"=w109) -> ()  [unwired: 2 in, 2 out]
          n87 = local write "AR.Visible"(w122) -> ()
          n88 = local write "AR.Color"(w125) -> ()
          n89 = local write "AR.Start Angle"(w124) -> ()
          n90 = Add(x=w134, y=w134) -> (x+y=w131:i16)
          n91 = Add(x=w136, y=w136) -> (x+y=w135:i16)
          n92 = local write "AR.End Radius"(w106) -> ()
          n93 = local write "AR.Name"(w127) -> ()
          n94 = property on="Cursor Info.Visible" class="Bool (strict)"("Disabled"=w131) -> ()  [unwired: 2 in, 2 out]
          n95 = property on="Cursor Info Position.Lock" class="Bool (strict)"("Disabled"=w135) -> ()  [unwired: 2 in, 2 out]
          n96 = Boolean To (0,1)(Boolean=w107) -> (0, 1=w108:i16)
          n97 = local write "AR.Fill Color"(w104) -> ()
          n98 = local write "AR.End Angle"(w123) -> ()
          n99 = Add(x=w108, y=w108) -> (x+y=w105:i16)
          n100 = control-ref of="AR.Style"() -> (w121:refnum<vi>)
          n101 = control-ref of="AR.Width"() -> (w118:refnum<vi>)
          n102 = property on="AR.Style" class="Clust (strict)"("Disabled"=w105) -> ()  [unwired: 2 in, 2 out]
          n103 = property on="AR.Visible" class="Bool (strict)"("Disabled"=w105) -> ()  [unwired: 2 in, 2 out]
          n104 = property on="AR.Width" class="Clust (strict)"("Disabled"=w105) -> ()  [unwired: 2 in, 2 out]
          n105 = property on="AR.Selector" class="Ring (strict)"("Disabled"=w105) -> ()  [unwired: 2 in, 2 out]
          n106 = property on="AR.Name" class="Str"("Disabled"=w105) -> ()  [unwired: 2 in, 2 out]
          n107 = property on="AR.Start Angle" class="DigNum (strict)"("Disabled"=w105) -> ()  [unwired: 2 in, 2 out]
          n108 = property on="AR.End Angle" class="DigNum (strict)"("Disabled"=w105) -> ()  [unwired: 2 in, 2 out]
          n109 = property on="AR.Start Radius" class="DigNum (strict)"("Disabled"=w105) -> ()  [unwired: 2 in, 2 out]
          n110 = property on="AR.End Radius" class="DigNum (strict)"("Disabled"=w105) -> ()  [unwired: 2 in, 2 out]
          n111 = property on="AR.Color" class="ColBox"("Disabled"=w105) -> ()  [unwired: 2 in, 2 out]
          n112 = property on="AR.Fill Color" class="ColBox"("Disabled"=w105) -> ()  [unwired: 2 in, 2 out]
          n113 = call <vilib>:"svx_Polar_Manage_Cluster.vi"("index"=w120, "Clust Refnum"=w121) -> ()  [unwired: 10 in]
          n114 = call <vilib>:"svx_Polar_Manage_Cluster.vi"("index"=w119, "Clust Refnum"=w118) -> ()  [unwired: 10 in]
        }
        frame #4 {
          n115 = property class="VI"(reference=w141, "Front Panel.Open"=TRUE ("Front Panel Window:Open")) -> ()  [unwired: 1 in, 2 out]
        }
      }
    }
    frame #1 {
      n116 = while {
        shift-right: [w168] -> w157
        shift-left: w158 -> [w176]
        tunnel: w156 -> [w175]
        shift-right: [w173] -> w154
        shift-left: w155 -> [w174]
        tunnel: w153 -> [w167]
        tunnel: w152 -> [w165]
        tunnel: w151 -> [w172]
        tunnel: w150 -> [w171]
        tunnel: w149 -> [w164]
        tunnel: w148 -> [w166]
        tunnel: w147 -> [w170]
        tunnel: [w170] -> w146
        tunnel: w145 -> [w163]
        shift-right: [w160] -> w143
        shift-left: w144 -> [w161]
        shift-right: [w159] -> _
        shift-left: w142 -> [w159]
        stop <- w177 stop-if-true
        n117 = event shown="[46] \"AR.Remove\": Value Change" {
          selector: _ -> [_ _ _ _ _ _ _ _ _ _ _ _ _ _ _ _ _ _ _ _ _ _ _ _ _ _ _ _ _ _ _ _ _ _ _ _ _ _ _ _ _ _ _ _ _ _ _ _ _ _ _ _ _ _ _ _ _ _]
          dyn-events: _ -> [_ _ _ _ _ _ _ _ _ _ _ _ _ _ _ _ _ _ _ _ _ _ _ _ _ _ _ _ _ _ _ _ _ _ _ _ _ _ _ _ _ _ _ _ _ _ _ _ _ _ _ _ _ _ _ _ _ _]
          timeout: _ -> [_ _ _ _ _ _ _ _ _ _ _ _ _ _ _ _ _ _ _ _ _ _ _ _ _ _ _ _ _ _ _ _ _ _ _ _ _ _ _ _ _ _ _ _ _ _ _ _ _ _ _ _ _ _ _ _ _ _]
          tunnel: [_ TRUE ("OK") TRUE ("OK") _ _ _ _ _ _ _ _ _ _ _ _ _ _ _ _ _ _ _ _ _ _ _ _ _ _ _ _ _ _ _ _ _ _ _ _ _ _ _ _ _ _ _ _ _ _ _ _ _ _ _ _ _ _ _] -> w177
          tunnel: [w180 w185 w194 w207 w215 w219 w225 w230 w236 w238 w242 w247 w255 w259 w271 w279 w284 w291 w293 w301 w306 w312 w315 w321 w334 w338 w341 w346 w351 w356 w360 w367 w372 w375 w380 w385 w402 w415 w428 w441 w454 w467 w481 w494 w502 w521 w561 w589 w597 w607 w615 w625 w635 w645 w655 w674 w692 w704] -> w169
          tunnel: w176 -> [w180 w185 _ w207 w215 w219 w225 w230 w236 w239 w244 w249 w256 w269 w273 w281 w287 w289 w295 w302 w309 w312 w316 w325 w334 w338 w342 w347 w352 w357 w361 w368 w373 w377 w382 w387 w403 w416 w429 w442 w455 w468 w480 w493 w504 w534 w572 w589 w600 w610 w618 w628 w638 w648 w658 w677 w695 w707]
          tunnel: w175 -> [_ _ w203 _ w214 w222 w228 w232 w234 _ _ _ _ _ _ _ _ _ _ _ _ _ _ _ w332 w336 _ _ _ _ _ _ _ _ _ _ _ _ _ _ _ _ _ _ _ _ _ _ _ _ _ _ _ _ _ _ _ _]
          tunnel: w174 -> [w179 w184 w195 w206 w211 w218 w227 w229 w235 w240 w245 w250 w254 w268 w277 w282 w286 w292 w297 w300 w310 w313 w318 w330 w333 w337 w343 w348 w353 w358 w363 w366 w371 w378 w383 w388 w404 w417 w430 w443 w456 w469 w482 w495 w505 w522 w562 w575 w598 w608 w616 w626 w636 w646 w656 w675 w693 w705]
          tunnel: [w179 w183 w195 w206 w211 w218 w227 w229 w235 w240 w245 w250 w254 w268 w277 w282 w286 w292 w297 w300 w310 w313 w318 w330 w333 w337 w343 w348 w353 w358 w363 w366 w371 w378 w383 w388 w404 w417 w430 w443 w456 w469 w482 w495 w505 w522 w562 w575 w598 w608 w616 w626 w636 w646 w656 w675 w693 w705] -> w173
          tunnel: w172 -> [_ w186 w191 _ _ _ _ _ _ _ _ _ _ _ _ _ _ _ _ _ _ _ _ _ _ _ _ _ _ _ _ _ _ _ _ _ _ _ _ _ _ _ _ _ _ _ _ _ _ _ _ _ _ _ _ _ _ _]
          tunnel: w165 -> [_ _ w192 _ _ _ _ _ _ _ _ _ _ _ _ _ _ _ _ _ _ _ _ w324 _ _ _ _ _ _ _ _ _ _ _ _ _ _ _ _ _ _ _ _ _ _ _ _ _ _ _ _ _ _ _ _ _ _]
          tunnel: w167 -> [_ _ w193 _ _ _ _ _ _ _ _ _ _ _ _ _ _ _ _ _ _ _ _ w322 _ _ _ _ _ _ _ _ _ _ _ _ _ _ _ _ _ _ _ _ _ _ _ _ _ _ _ _ _ _ _ _ _ _]
          tunnel: w171 -> [_ _ w204 _ _ _ _ _ _ _ _ _ _ _ _ _ _ _ _ _ _ _ _ _ _ _ _ _ _ _ _ _ _ _ _ _ _ _ _ _ _ _ _ _ _ _ _ _ _ _ _ _ _ _ _ _ _ _]
          tunnel: w164 -> [_ _ w190 _ _ _ _ _ _ _ _ _ _ _ _ _ _ _ _ _ _ _ _ _ _ _ _ _ _ _ _ _ _ _ _ _ _ _ _ _ _ _ _ _ _ _ _ _ _ _ _ _ _ _ _ _ _ _]
          tunnel: w166 -> [_ _ w189 _ _ _ _ _ _ _ _ _ _ _ _ _ _ _ _ _ _ _ _ _ _ _ _ _ _ _ _ _ _ _ _ _ _ _ _ _ _ _ _ _ _ _ _ _ _ _ _ _ _ _ _ _ _ _]
          tunnel: w170 -> [_ _ _ _ _ _ _ _ _ _ _ _ _ _ _ _ _ _ _ _ _ _ _ _ _ _ _ _ _ _ _ _ _ _ _ _ _ _ _ _ _ _ _ _ _ _ _ _ _ _ _ _ _ _ _ _ _ _]
          tunnel: w163 -> [_ _ _ _ _ _ _ _ _ _ _ _ _ _ _ _ _ _ _ _ _ _ _ _ _ _ _ _ _ _ _ _ _ _ _ _ _ _ _ _ _ _ _ _ _ _ _ _ _ _ _ _ _ _ _ _ _ _]
          tunnel: [w178 _ w188 _ _ _ _ _ _ w237 w243 w248 w252 w257 w270 w278 w283 w288 w294 w298 w305 _ w314 w319 _ _ w339 w344 w349 w354 w359 w364 w369 w374 w379 w384 w397 w410 w423 w436 w449 w462 w475 w488 w501 w506 w538 _ w590 w604 w614 w624 w634 w644 w654 w664 w682 _] -> w162
          event Timeout {
            w178 = T15[] [] items=["[Data] Update Data", "[Scale] Update Polar Scale", "[Scale] Autoscale", "[Legend] Update Legend", "[Cursor] Cursor Release", "[Pane] Change Minimum Size", "[Annt] Upodate Annotation", "[Plot] Appearance", "[Cursor] Visibility", "[Cursor] Appearance", "[Cursor] Index", "[Scale] MagnitudeVisibility", "[Scale] PhaseVisibility", "[Scale] PhaseAppearance", "[Scale] MagnitudeApperance", "[Plot] AcceptanceRegion", "[Scale] RangeChange", "[Marker] Appearance", "[Marker] List", "[Marker] Visibility", "[Legend] Visibility", "[Legend] Color", "[Data] Index", "[Legend] Update String", "[Cursor] Trigger Event", "[Scale] Trigger Event", "[Data] Clear Graph"] ("To Do")
            n118 = event-data() -> ()  [unwired: 1 in, 1 out]
          }
          event "OK": Value Change {
            n119 = event-data() -> ()  [unwired: 1 in, 1 out]
            n120 = Not Equal?(x=w185, y=w186) -> (x != y?=w182:bool)
            n121 = Bundle By Name(cluster=w184, "Action Name"="Property Page Edits", "State Changed?"=w182) -> (w183:T3)
          }
          event Panel Close; "Cancel": Value Change {
            w188 = T15[] [enum."[Data] Update Data", enum."[Scale] Autoscale", enum."[Scale] Update Polar Scale", enum."[Legend] Update Legend"] items=["[Data] Update Data", "[Scale] Update Polar Scale", "[Scale] Autoscale", "[Legend] Update Legend", "[Cursor] Cursor Release", "[Pane] Change Minimum Size", "[Annt] Upodate Annotation", "[Plot] Appearance", "[Cursor] Visibility", "[Cursor] Appearance", "[Cursor] Index", "[Scale] MagnitudeVisibility", "[Scale] PhaseVisibility", "[Scale] PhaseAppearance", "[Scale] MagnitudeApperance", "[Plot] AcceptanceRegion", "[Scale] RangeChange", "[Marker] Appearance", "[Marker] List", "[Marker] Visibility", "[Legend] Visibility", "[Legend] Color", "[Data] Index", "[Legend] Update String", "[Cursor] Trigger Event", "[Scale] Trigger Event", "[Data] Clear Graph"] ("To Do")
            n122 = event-data() -> ()  [unwired: 1 in, 3 out]
            n123 = call <vilib>:"svx_Polar_Property_Dialog_Cancel.vi"("Plot Legend ref in"=w189, "Cursor Info ref in"=w190, "z scale graph ref in"=w192, "Polar Plot ref in"=w193, "State in"=w191) -> ("State out"=w194:T4)  [unwired: 6 in]
            n124 = Unbundle(w204) -> ("Label.Text"=w202:string, "Caption.Text"=w201:string, "Label.Visible"=w200:bool, "Caption.Visible"=w199:bool, "Disabled"=w198:u8, "Desc"=w197:string, "TipStrip"=w196:string)
            n125 = property class="Ctl"(reference=w203, "Label.Text"=w202, "Caption.Text"=w201, "Label.Visible"=w200, "Caption.Visible"=w199, "Disabled"=w198, "Desc"=w197, "TipStrip"=w196) -> ()  [unwired: 1 in, 2 out]
          }
          event "Help": Value Change {
            n126 = event-data() -> ()  [unwired: 1 in, 1 out]
            n127 = Control Online Help(2:path "<helpdir>/sndvibtk.chm" ("Path to the help file"), 3:"Polar_Plot_DB.html" ("String to search for"), 4:enum16{"Contents", "Key", "Close"}."Key" ("Operation")) -> ()  [unwired: 1 in, 1 out]
          }
          event "Label.Visible": Value Change {
            n128 = event-data() -> ("NewVal"=w213:bool)  [unwired: 1 in]
            n129 = Select(t=u8 0 ("Disabled"), s=w213, f=u8 2 ("Disabled")) -> (s? t:f=w212:u8)
            n130 = property class="Ctl"(reference=w214, "Label.Visible"=w213) -> ()  [unwired: 1 in, 2 out]
            n131 = property on="Label.Text" class="Str"("Disabled"=w212) -> ()  [unwired: 2 in, 2 out]
          }
          event "Caption.Visible": Value Change {
            n132 = event-data() -> ("NewVal"=w221:bool)  [unwired: 1 in]
            n133 = Select(t=u8 0 ("Disabled"), s=w221, f=u8 2 ("Disabled")) -> (s? t:f=w220:u8)
            n134 = property class="Ctl"(reference=w222, "Caption.Visible"=w221) -> ()  [unwired: 1 in, 2 out]
            n135 = property on="Caption.Text" class="Str"("Disabled"=w220) -> ()  [unwired: 2 in, 2 out]
          }
          event "Caption.Text": Value Change {
            n136 = event-data() -> ("NewVal"=w226:string)  [unwired: 1 in]
            n137 = property class="Ctl"(reference=w228, "Caption.Text"=w226) -> ()  [unwired: 1 in, 2 out]
          }
          event "Label.Text": Value Change {
            n138 = event-data() -> ("NewVal"=w231:string)  [unwired: 1 in]
            n139 = property class="Ctl"(reference=w232, "Label.Text"=w231) -> ()  [unwired: 1 in, 2 out]
          }
          event "Enable State": Value Change {
            n140 = event-data() -> ("NewVal"=w233:T8)  [unwired: 1 in]
            n141 = property class="Ctl"(reference=w234, "Disabled"=w233) -> ()  [unwired: 1 in, 2 out]
          }
          event "Arrow.Color": Value Change {
            w237 = T15[] [enum."[Scale] Update Polar Scale"] items=["[Data] Update Data", "[Scale] Update Polar Scale", "[Scale] Autoscale", "[Legend] Update Legend", "[Cursor] Cursor Release", "[Pane] Change Minimum Size", "[Annt] Upodate Annotation", "[Plot] Appearance", "[Cursor] Visibility", "[Cursor] Appearance", "[Cursor] Index", "[Scale] MagnitudeVisibility", "[Scale] PhaseVisibility", "[Scale] PhaseAppearance", "[Scale] MagnitudeApperance", "[Plot] AcceptanceRegion", "[Scale] RangeChange", "[Marker] Appearance", "[Marker] List", "[Marker] Visibility", "[Legend] Visibility", "[Legend] Color", "[Data] Index", "[Legend] Update String", "[Cursor] Trigger Event", "[Scale] Trigger Event", "[Data] Clear Graph"] ("To Do")
            n142 = event-data() -> ("NewVal"=w241:u32)  [unwired: 1 in]
            n143 = Bundle By Name(cluster=w239, "Color settings.Arrow color"=w241) -> (w238:T4)
          }
          event "Phase Grid.Color": Value Change {
            w243 = T15[] [enum."[Scale] PhaseAppearance"] items=["[Data] Update Data", "[Scale] Update Polar Scale", "[Scale] Autoscale", "[Legend] Update Legend", "[Cursor] Cursor Release", "[Pane] Change Minimum Size", "[Annt] Upodate Annotation", "[Plot] Appearance", "[Cursor] Visibility", "[Cursor] Appearance", "[Cursor] Index", "[Scale] MagnitudeVisibility", "[Scale] PhaseVisibility", "[Scale] PhaseAppearance", "[Scale] MagnitudeApperance", "[Plot] AcceptanceRegion", "[Scale] RangeChange", "[Marker] Appearance", "[Marker] List", "[Marker] Visibility", "[Legend] Visibility", "[Legend] Color", "[Data] Index", "[Legend] Update String", "[Cursor] Trigger Event", "[Scale] Trigger Event", "[Data] Clear Graph"] ("To Do")
            n144 = event-data() -> ("NewVal"=w246:u32)  [unwired: 1 in]
            n145 = Bundle By Name(cluster=w244, "Color settings.Phase grid"=w246) -> (w242:T4)
          }
          event "Phase Scale Marker Text.Color": Value Change {
            w248 = T15[] [enum."[Scale] PhaseAppearance"] items=["[Data] Update Data", "[Scale] Update Polar Scale", "[Scale] Autoscale", "[Legend] Update Legend", "[Cursor] Cursor Release", "[Pane] Change Minimum Size", "[Annt] Upodate Annotation", "[Plot] Appearance", "[Cursor] Visibility", "[Cursor] Appearance", "[Cursor] Index", "[Scale] MagnitudeVisibility", "[Scale] PhaseVisibility", "[Scale] PhaseAppearance", "[Scale] MagnitudeApperance", "[Plot] AcceptanceRegion", "[Scale] RangeChange", "[Marker] Appearance", "[Marker] List", "[Marker] Visibility", "[Legend] Visibility", "[Legend] Color", "[Data] Index", "[Legend] Update String", "[Cursor] Trigger Event", "[Scale] Trigger Event", "[Data] Clear Graph"] ("To Do")
            n146 = event-data() -> ("NewVal"=w251:u32)  [unwired: 1 in]
            n147 = Bundle By Name(cluster=w249, "Color settings.Phase scale marker text"=w251) -> (w247:T4)
          }
          event "Marker.Color": Value Change {
            w252 = T15[] [enum."[Marker] Appearance"] items=["[Data] Update Data", "[Scale] Update Polar Scale", "[Scale] Autoscale", "[Legend] Update Legend", "[Cursor] Cursor Release", "[Pane] Change Minimum Size", "[Annt] Upodate Annotation", "[Plot] Appearance", "[Cursor] Visibility", "[Cursor] Appearance", "[Cursor] Index", "[Scale] MagnitudeVisibility", "[Scale] PhaseVisibility", "[Scale] PhaseAppearance", "[Scale] MagnitudeApperance", "[Plot] AcceptanceRegion", "[Scale] RangeChange", "[Marker] Appearance", "[Marker] List", "[Marker] Visibility", "[Legend] Visibility", "[Legend] Color", "[Data] Index", "[Legend] Update String", "[Cursor] Trigger Event", "[Scale] Trigger Event", "[Data] Clear Graph"] ("To Do")
            n148 = event-data() -> ("NewVal"=w253:u32)  [unwired: 1 in]
            n149 = Bundle By Name(cluster=w256, "Marker color"=w253) -> (w255:T4)
          }
          event "Cursor.Visible": Value Change {
            w257 = T15[] [enum."[Cursor] Visibility", enum."[Cursor] Cursor Release"] items=["[Data] Update Data", "[Scale] Update Polar Scale", "[Scale] Autoscale", "[Legend] Update Legend", "[Cursor] Cursor Release", "[Pane] Change Minimum Size", "[Annt] Upodate Annotation", "[Plot] Appearance", "[Cursor] Visibility", "[Cursor] Appearance", "[Cursor] Index", "[Scale] MagnitudeVisibility", "[Scale] PhaseVisibility", "[Scale] PhaseAppearance", "[Scale] MagnitudeApperance", "[Plot] AcceptanceRegion", "[Scale] RangeChange", "[Marker] Appearance", "[Marker] List", "[Marker] Visibility", "[Legend] Visibility", "[Legend] Color", "[Data] Index", "[Legend] Update String", "[Cursor] Trigger Event", "[Scale] Trigger Event", "[Data] Clear Graph"] ("To Do")
            n150 = event-data() -> ("NewVal"=w258:bool)  [unwired: 1 in]
            n151 = local read "Cursor Info.Visible"() -> (w265:bool)
            n152 = Bundle By Name(cluster=w269, "Cursor:Visible"=w258) -> (w259:T4)
            n153 = And(x=w258, y=w265) -> (x .and. y?=w261:bool)
            n154 = Not(x=w258) -> (.not. x?=w262:bool)
            n155 = Not(x=w261) -> (.not. x?=w263:bool)
            n156 = Boolean To (0,1)(Boolean=w262) -> (0, 1=w267:i16)
            n157 = Boolean To (0,1)(Boolean=w263) -> (0, 1=w264:i16)
            n158 = Add(x=w267, y=w267) -> (x+y=w266:i16)
            n159 = Add(x=w264, y=w264) -> (x+y=w260:i16)
            n160 = property on="Cursor Info.Visible" class="Bool (strict)"("Disabled"=w266) -> ()  [unwired: 2 in, 2 out]
            n161 = property on="Cursor Info Position.Lock" class="Bool (strict)"("Disabled"=w260) -> ()  [unwired: 2 in, 2 out]
          }
          event "Cursor Info.Visible": Value Change {
            w270 = T15[] [enum."[Cursor] Visibility", enum."[Cursor] Cursor Release"] items=["[Data] Update Data", "[Scale] Update Polar Scale", "[Scale] Autoscale", "[Legend] Update Legend", "[Cursor] Cursor Release", "[Pane] Change Minimum Size", "[Annt] Upodate Annotation", "[Plot] Appearance", "[Cursor] Visibility", "[Cursor] Appearance", "[Cursor] Index", "[Scale] MagnitudeVisibility", "[Scale] PhaseVisibility", "[Scale] PhaseAppearance", "[Scale] MagnitudeApperance", "[Plot] AcceptanceRegion", "[Scale] RangeChange", "[Marker] Appearance", "[Marker] List", "[Marker] Visibility", "[Legend] Visibility", "[Legend] Color", "[Data] Index", "[Legend] Update String", "[Cursor] Trigger Event", "[Scale] Trigger Event", "[Data] Clear Graph"] ("To Do")
            n162 = event-data() -> ("NewVal"=w272:bool)  [unwired: 1 in]
            n163 = Bundle By Name(cluster=w273, "CursorName:Visible"=w272) -> (w271:T4)
            n164 = Not(x=w272) -> (.not. x?=w276:bool)
            n165 = Boolean To (0,1)(Boolean=w276) -> (0, 1=w275:i16)
            n166 = Add(x=w275, y=w275) -> (x+y=w274:i16)
            n167 = property on="Cursor Info Position.Lock" class="Bool (strict)"("Disabled"=w274) -> ()  [unwired: 2 in, 2 out]
          }
          event "Cursor Info Position.Lock": Value Change {
            w278 = T15[] [enum."[Cursor] Visibility", enum."[Cursor] Cursor Release"] items=["[Data] Update Data", "[Scale] Update Polar Scale", "[Scale] Autoscale", "[Legend] Update Legend", "[Cursor] Cursor Release", "[Pane] Change Minimum Size", "[Annt] Upodate Annotation", "[Plot] Appearance", "[Cursor] Visibility", "[Cursor] Appearance", "[Cursor] Index", "[Scale] MagnitudeVisibility", "[Scale] PhaseVisibility", "[Scale] PhaseAppearance", "[Scale] MagnitudeApperance", "[Plot] AcceptanceRegion", "[Scale] RangeChange", "[Marker] Appearance", "[Marker] List", "[Marker] Visibility", "[Legend] Visibility", "[Legend] Color", "[Data] Index", "[Legend] Update String", "[Cursor] Trigger Event", "[Scale] Trigger Event", "[Data] Clear Graph"] ("To Do")
            n168 = event-data() -> ("NewVal"=w280:bool)  [unwired: 1 in]
            n169 = Bundle By Name(cluster=w281, "Lock Cursor Info Position"=w280) -> (w279:T4)
          }
          event "Magnitude Scale.Visible": Value Change {
            w283 = T15[] [enum."[Scale] MagnitudeVisibility"] items=["[Data] Update Data", "[Scale] Update Polar Scale", "[Scale] Autoscale", "[Legend] Update Legend", "[Cursor] Cursor Release", "[Pane] Change Minimum Size", "[Annt] Upodate Annotation", "[Plot] Appearance", "[Cursor] Visibility", "[Cursor] Appearance", "[Cursor] Index", "[Scale] MagnitudeVisibility", "[Scale] PhaseVisibility", "[Scale] PhaseAppearance", "[Scale] MagnitudeApperance", "[Plot] AcceptanceRegion", "[Scale] RangeChange", "[Marker] Appearance", "[Marker] List", "[Marker] Visibility", "[Legend] Visibility", "[Legend] Color", "[Data] Index", "[Legend] Update String", "[Cursor] Trigger Event", "[Scale] Trigger Event", "[Data] Clear Graph"] ("To Do")
            n170 = event-data() -> ("NewVal"=w285:bool)  [unwired: 1 in]
            n171 = Bundle By Name(cluster=w287, "MagnitudeScale:Visible"=w285) -> (w284:T4)
          }
          event "Magnitude Scale Label.Visible": Value Change {
            w288 = T15[] [enum."[Scale] MagnitudeVisibility"] items=["[Data] Update Data", "[Scale] Update Polar Scale", "[Scale] Autoscale", "[Legend] Update Legend", "[Cursor] Cursor Release", "[Pane] Change Minimum Size", "[Annt] Upodate Annotation", "[Plot] Appearance", "[Cursor] Visibility", "[Cursor] Appearance", "[Cursor] Index", "[Scale] MagnitudeVisibility", "[Scale] PhaseVisibility", "[Scale] PhaseAppearance", "[Scale] MagnitudeApperance", "[Plot] AcceptanceRegion", "[Scale] RangeChange", "[Marker] Appearance", "[Marker] List", "[Marker] Visibility", "[Legend] Visibility", "[Legend] Color", "[Data] Index", "[Legend] Update String", "[Cursor] Trigger Event", "[Scale] Trigger Event", "[Data] Clear Graph"] ("To Do")
            n172 = event-data() -> ("NewVal"=w290:bool)  [unwired: 1 in]
            n173 = Bundle By Name(cluster=w289, "MagnitudeScaleLabel:Visible"=w290) -> (w291:T4)
          }
          event "Phase Scale.Visible": Value Change {
            w294 = T15[] [enum."[Scale] PhaseVisibility"] items=["[Data] Update Data", "[Scale] Update Polar Scale", "[Scale] Autoscale", "[Legend] Update Legend", "[Cursor] Cursor Release", "[Pane] Change Minimum Size", "[Annt] Upodate Annotation", "[Plot] Appearance", "[Cursor] Visibility", "[Cursor] Appearance", "[Cursor] Index", "[Scale] MagnitudeVisibility", "[Scale] PhaseVisibility", "[Scale] PhaseAppearance", "[Scale] MagnitudeApperance", "[Plot] AcceptanceRegion", "[Scale] RangeChange", "[Marker] Appearance", "[Marker] List", "[Marker] Visibility", "[Legend] Visibility", "[Legend] Color", "[Data] Index", "[Legend] Update String", "[Cursor] Trigger Event", "[Scale] Trigger Event", "[Data] Clear Graph"] ("To Do")
            n174 = event-data() -> ("NewVal"=w296:bool)  [unwired: 1 in]
            n175 = Bundle By Name(cluster=w295, "PhaseScale:Visible"=w296) -> (w293:T4)
          }
          event "Magnitude.Text": Value Change {
            w298 = T15[] [enum."[Scale] MagnitudeApperance"] items=["[Data] Update Data", "[Scale] Update Polar Scale", "[Scale] Autoscale", "[Legend] Update Legend", "[Cursor] Cursor Release", "[Pane] Change Minimum Size", "[Annt] Upodate Annotation", "[Plot] Appearance", "[Cursor] Visibility", "[Cursor] Appearance", "[Cursor] Index", "[Scale] MagnitudeVisibility", "[Scale] PhaseVisibility", "[Scale] PhaseAppearance", "[Scale] MagnitudeApperance", "[Plot] AcceptanceRegion", "[Scale] RangeChange", "[Marker] Appearance", "[Marker] List", "[Marker] Visibility", "[Legend] Visibility", "[Legend] Color", "[Data] Index", "[Legend] Update String", "[Cursor] Trigger Event", "[Scale] Trigger Event", "[Data] Clear Graph"] ("To Do")
            n176 = event-data() -> ("NewVal"=w299:string)  [unwired: 1 in]
            n177 = Bundle By Name(cluster=w302, "Magnitude scale name"=w299) -> (w301:T4)
          }
          event "Magnitude.Scale Fit": Value Change {
            w305 = T15[] [enum."[Scale] Autoscale"] items=["[Data] Update Data", "[Scale] Update Polar Scale", "[Scale] Autoscale", "[Legend] Update Legend", "[Cursor] Cursor Release", "[Pane] Change Minimum Size", "[Annt] Upodate Annotation", "[Plot] Appearance", "[Cursor] Visibility", "[Cursor] Appearance", "[Cursor] Index", "[Scale] MagnitudeVisibility", "[Scale] PhaseVisibility", "[Scale] PhaseAppearance", "[Scale] MagnitudeApperance", "[Plot] AcceptanceRegion", "[Scale] RangeChange", "[Marker] Appearance", "[Marker] List", "[Marker] Visibility", "[Legend] Visibility", "[Legend] Color", "[Data] Index", "[Legend] Update String", "[Cursor] Trigger Event", "[Scale] Trigger Event", "[Data] Clear Graph"] ("To Do")
            n178 = event-data() -> ("NewVal"=w303:bool)  [unwired: 1 in]
            n179 = Bundle By Name(cluster=w309, "Autoscale"=w303) -> (w306:T4)
            n180 = property on="update maximum value" class="Bool (strict)"("Val(Sgnl)"=w303) -> ()  [unwired: 2 in, 2 out]
            n181 = Select(t=u8 2 ("Disabled"), s=w303, f=u8 0 ("Disabled")) -> (s? t:f=w307:u8)
            n182 = property on="Magnitude Range:Maximum" class="DigNum (strict)"("Disabled"=w307) -> ()  [unwired: 2 in, 2 out]
          }
          event "update maximum value": Value Change {
            n183 = event-data() -> ()  [unwired: 1 in, 6 out]
            n184 = Unbundle By Name(w312) -> ("Scale range.Maximum"=w311:dbl)
            n185 = local write "Magnitude Range:Maximum"(w311) -> ()
          }
          event "Magnitude Range:Maximum": Value Change {
            w314 = T15[] [enum."[Scale] RangeChange"] items=["[Data] Update Data", "[Scale] Update Polar Scale", "[Scale] Autoscale", "[Legend] Update Legend", "[Cursor] Cursor Release", "[Pane] Change Minimum Size", "[Annt] Upodate Annotation", "[Plot] Appearance", "[Cursor] Visibility", "[Cursor] Appearance", "[Cursor] Index", "[Scale] MagnitudeVisibility", "[Scale] PhaseVisibility", "[Scale] PhaseAppearance", "[Scale] MagnitudeApperance", "[Plot] AcceptanceRegion", "[Scale] RangeChange", "[Marker] Appearance", "[Marker] List", "[Marker] Visibility", "[Legend] Visibility", "[Legend] Color", "[Data] Index", "[Legend] Update String", "[Cursor] Trigger Event", "[Scale] Trigger Event", "[Data] Clear Graph"] ("To Do")
            n186 = event-data() -> ("NewVal"=w317:dbl)  [unwired: 1 in]
            n187 = Bundle By Name(cluster=w316, "Scale range.Maximum"=w317) -> (w315:T4)
          }
          event "Type", "Digits", "Hide trailing zeros", "Precision Type": Value Change {
            w319 = T15[] [enum."[Scale] Update Polar Scale"] items=["[Data] Update Data", "[Scale] Update Polar Scale", "[Scale] Autoscale", "[Legend] Update Legend", "[Cursor] Cursor Release", "[Pane] Change Minimum Size", "[Annt] Upodate Annotation", "[Plot] Appearance", "[Cursor] Visibility", "[Cursor] Appearance", "[Cursor] Index", "[Scale] MagnitudeVisibility", "[Scale] PhaseVisibility", "[Scale] PhaseAppearance", "[Scale] MagnitudeApperance", "[Plot] AcceptanceRegion", "[Scale] RangeChange", "[Marker] Appearance", "[Marker] List", "[Marker] Visibility", "[Legend] Visibility", "[Legend] Color", "[Data] Index", "[Legend] Update String", "[Cursor] Trigger Event", "[Scale] Trigger Event", "[Data] Clear Graph"] ("To Do")
            n188 = event-data() -> ()  [unwired: 1 in, 1 out]
            n189 = call <vilib>:"svx_Polar_To_FString.vi"("trailing zeros"="Hide trailing zeros", "Precision Type"="Precision Type", "Digits"="Digits", "Type"="Type") -> ("format string"=w323:string)  [unwired: 7 in]
            n190 = Bundle By Name(cluster=w325, "Magnitude scale format string"=w323) -> (w321:T4)
            n191 = property class="XYGraph (strict)"(reference=w324, "YScale.FormatString"=w323) -> (reference out=w320:refnum<vi>)  [unwired: 1 in, 1 out]
            n192 = call <vilib>:"svx_Polar_Align_Plot_Area.vi"("z scale graph ref in"=w320, "Polar Plot ref in"=w322) -> ()  [unwired: 8 in, 2 out]
          }
          event "Description": Value Change {
            n193 = event-data() -> ("NewVal"=w331:string)  [unwired: 1 in]
            n194 = property class="Ctl"(reference=w332, "Desc"=w331) -> ()  [unwired: 1 in, 2 out]
          }
          event "Tip strip": Value Change {
            n195 = event-data() -> ("NewVal"=w335:string)  [unwired: 1 in]
            n196 = property class="Ctl"(reference=w336, "TipStrip"=w335) -> ()  [unwired: 1 in, 2 out]
          }
          event "Line.Color": Value Change {
            w339 = T15[] [enum."[Plot] Appearance"] items=["[Data] Update Data", "[Scale] Update Polar Scale", "[Scale] Autoscale", "[Legend] Update Legend", "[Cursor] Cursor Release", "[Pane] Change Minimum Size", "[Annt] Upodate Annotation", "[Plot] Appearance", "[Cursor] Visibility", "[Cursor] Appearance", "[Cursor] Index", "[Scale] MagnitudeVisibility", "[Scale] PhaseVisibility", "[Scale] PhaseAppearance", "[Scale] MagnitudeApperance", "[Plot] AcceptanceRegion", "[Scale] RangeChange", "[Marker] Appearance", "[Marker] List", "[Marker] Visibility", "[Legend] Visibility", "[Legend] Color", "[Data] Index", "[Legend] Update String", "[Cursor] Trigger Event", "[Scale] Trigger Event", "[Data] Clear Graph"] ("To Do")
            n197 = event-data() -> ("NewVal"=w340:u32)  [unwired: 1 in]
            n198 = Bundle By Name(cluster=w342, "Line color"=w340) -> (w341:T4)
          }
          event "Point/Fill.Color": Value Change {
            w344 = T15[] [enum."[Plot] Appearance"] items=["[Data] Update Data", "[Scale] Update Polar Scale", "[Scale] Autoscale", "[Legend] Update Legend", "[Cursor] Cursor Release", "[Pane] Change Minimum Size", "[Annt] Upodate Annotation", "[Plot] Appearance", "[Cursor] Visibility", "[Cursor] Appearance", "[Cursor] Index", "[Scale] MagnitudeVisibility", "[Scale] PhaseVisibility", "[Scale] PhaseAppearance", "[Scale] MagnitudeApperance", "[Plot] AcceptanceRegion", "[Scale] RangeChange", "[Marker] Appearance", "[Marker] List", "[Marker] Visibility", "[Legend] Visibility", "[Legend] Color", "[Data] Index", "[Legend] Update String", "[Cursor] Trigger Event", "[Scale] Trigger Event", "[Data] Clear Graph"] ("To Do")
            n199 = event-data() -> ("NewVal"=w345:u32)  [unwired: 1 in]
            n200 = Bundle By Name(cluster=w347, "Point/fill color"=w345) -> (w346:T4)
          }
          event "Cursor.Color": Value Change {
            w349 = T15[] [enum."[Cursor] Appearance"] items=["[Data] Update Data", "[Scale] Update Polar Scale", "[Scale] Autoscale", "[Legend] Update Legend", "[Cursor] Cursor Release", "[Pane] Change Minimum Size", "[Annt] Upodate Annotation", "[Plot] Appearance", "[Cursor] Visibility", "[Cursor] Appearance", "[Cursor] Index", "[Scale] MagnitudeVisibility", "[Scale] PhaseVisibility", "[Scale] PhaseAppearance", "[Scale] MagnitudeApperance", "[Plot] AcceptanceRegion", "[Scale] RangeChange", "[Marker] Appearance", "[Marker] List", "[Marker] Visibility", "[Legend] Visibility", "[Legend] Color", "[Data] Index", "[Legend] Update String", "[Cursor] Trigger Event", "[Scale] Trigger Event", "[Data] Clear Graph"] ("To Do")
            n201 = event-data() -> ("NewVal"=w350:u32)  [unwired: 1 in]
            n202 = Bundle By Name(cluster=w352, "Cursor color"=w350) -> (w351:T4)
          }
          event "Magnitude Scale Marker Text.Color": Value Change {
            w354 = T15[] [enum."[Scale] MagnitudeApperance"] items=["[Data] Update Data", "[Scale] Update Polar Scale", "[Scale] Autoscale", "[Legend] Update Legend", "[Cursor] Cursor Release", "[Pane] Change Minimum Size", "[Annt] Upodate Annotation", "[Plot] Appearance", "[Cursor] Visibility", "[Cursor] Appearance", "[Cursor] Index", "[Scale] MagnitudeVisibility", "[Scale] PhaseVisibility", "[Scale] PhaseAppearance", "[Scale] MagnitudeApperance", "[Plot] AcceptanceRegion", "[Scale] RangeChange", "[Marker] Appearance", "[Marker] List", "[Marker] Visibility", "[Legend] Visibility", "[Legend] Color", "[Data] Index", "[Legend] Update String", "[Cursor] Trigger Event", "[Scale] Trigger Event", "[Data] Clear Graph"] ("To Do")
            n203 = event-data() -> ("NewVal"=w355:u32)  [unwired: 1 in]
            n204 = Bundle By Name(cluster=w357, "Magnitude scale marker color"=w355) -> (w356:T4)
          }
          event "Background.Color": Value Change {
            w359 = T15[] [enum."[Plot] Appearance"] items=["[Data] Update Data", "[Scale] Update Polar Scale", "[Scale] Autoscale", "[Legend] Update Legend", "[Cursor] Cursor Release", "[Pane] Change Minimum Size", "[Annt] Upodate Annotation", "[Plot] Appearance", "[Cursor] Visibility", "[Cursor] Appearance", "[Cursor] Index", "[Scale] MagnitudeVisibility", "[Scale] PhaseVisibility", "[Scale] PhaseAppearance", "[Scale] MagnitudeApperance", "[Plot] AcceptanceRegion", "[Scale] RangeChange", "[Marker] Appearance", "[Marker] List", "[Marker] Visibility", "[Legend] Visibility", "[Legend] Color", "[Data] Index", "[Legend] Update String", "[Cursor] Trigger Event", "[Scale] Trigger Event", "[Data] Clear Graph"] ("To Do")
            n205 = event-data() -> ("NewVal"=w362:u32)  [unwired: 1 in]
            n206 = Bundle By Name(cluster=w361, "Background color"=w362) -> (w360:T4)
          }
          event "Plot Legend Background.Color": Value Change {
            w364 = T15[] [enum."[Legend] Color"] items=["[Data] Update Data", "[Scale] Update Polar Scale", "[Scale] Autoscale", "[Legend] Update Legend", "[Cursor] Cursor Release", "[Pane] Change Minimum Size", "[Annt] Upodate Annotation", "[Plot] Appearance", "[Cursor] Visibility", "[Cursor] Appearance", "[Cursor] Index", "[Scale] MagnitudeVisibility", "[Scale] PhaseVisibility", "[Scale] PhaseAppearance", "[Scale] MagnitudeApperance", "[Plot] AcceptanceRegion", "[Scale] RangeChange", "[Marker] Appearance", "[Marker] List", "[Marker] Visibility", "[Legend] Visibility", "[Legend] Color", "[Data] Index", "[Legend] Update String", "[Cursor] Trigger Event", "[Scale] Trigger Event", "[Data] Clear Graph"] ("To Do")
            n207 = event-data() -> ("NewVal"=w365:u32)  [unwired: 1 in]
            n208 = Bundle By Name(cluster=w368, "Legend BG color"=w365) -> (w367:T4)
          }
          event "Plot Legend Font.Color": Value Change {
            w369 = T15[] [enum."[Legend] Color"] items=["[Data] Update Data", "[Scale] Update Polar Scale", "[Scale] Autoscale", "[Legend] Update Legend", "[Cursor] Cursor Release", "[Pane] Change Minimum Size", "[Annt] Upodate Annotation", "[Plot] Appearance", "[Cursor] Visibility", "[Cursor] Appearance", "[Cursor] Index", "[Scale] MagnitudeVisibility", "[Scale] PhaseVisibility", "[Scale] PhaseAppearance", "[Scale] MagnitudeApperance", "[Plot] AcceptanceRegion", "[Scale] RangeChange", "[Marker] Appearance", "[Marker] List", "[Marker] Visibility", "[Legend] Visibility", "[Legend] Color", "[Data] Index", "[Legend] Update String", "[Cursor] Trigger Event", "[Scale] Trigger Event", "[Data] Clear Graph"] ("To Do")
            n209 = event-data() -> ("NewVal"=w370:u32)  [unwired: 1 in]
            n210 = Bundle By Name(cluster=w373, "Legend font color"=w370) -> (w372:T4)
          }
          event "Magnitude Major Grid.Color": Value Change {
            w374 = T15[] [enum."[Scale] MagnitudeApperance"] items=["[Data] Update Data", "[Scale] Update Polar Scale", "[Scale] Autoscale", "[Legend] Update Legend", "[Cursor] Cursor Release", "[Pane] Change Minimum Size", "[Annt] Upodate Annotation", "[Plot] Appearance", "[Cursor] Visibility", "[Cursor] Appearance", "[Cursor] Index", "[Scale] MagnitudeVisibility", "[Scale] PhaseVisibility", "[Scale] PhaseAppearance", "[Scale] MagnitudeApperance", "[Plot] AcceptanceRegion", "[Scale] RangeChange", "[Marker] Appearance", "[Marker] List", "[Marker] Visibility", "[Legend] Visibility", "[Legend] Color", "[Data] Index", "[Legend] Update String", "[Cursor] Trigger Event", "[Scale] Trigger Event", "[Data] Clear Graph"] ("To Do")
            n211 = event-data() -> ("NewVal"=w376:u32)  [unwired: 1 in]
            n212 = Bundle By Name(cluster=w377, "Color settings.Magnitude major grid"=w376) -> (w375:T4)
          }
          event "Magnitude Minor Grid.Color": Value Change {
            w379 = T15[] [enum."[Scale] MagnitudeApperance"] items=["[Data] Update Data", "[Scale] Update Polar Scale", "[Scale] Autoscale", "[Legend] Update Legend", "[Cursor] Cursor Release", "[Pane] Change Minimum Size", "[Annt] Upodate Annotation", "[Plot] Appearance", "[Cursor] Visibility", "[Cursor] Appearance", "[Cursor] Index", "[Scale] MagnitudeVisibility", "[Scale] PhaseVisibility", "[Scale] PhaseAppearance", "[Scale] MagnitudeApperance", "[Plot] AcceptanceRegion", "[Scale] RangeChange", "[Marker] Appearance", "[Marker] List", "[Marker] Visibility", "[Legend] Visibility", "[Legend] Color", "[Data] Index", "[Legend] Update String", "[Cursor] Trigger Event", "[Scale] Trigger Event", "[Data] Clear Graph"] ("To Do")
            n213 = event-data() -> ("NewVal"=w381:u32)  [unwired: 1 in]
            n214 = Bundle By Name(cluster=w382, "Color settings.Magnitude minor grid"=w381) -> (w380:T4)
          }
          event "Plot.Line Style": Value Change {
            w384 = T15[] [enum."[Plot] Appearance"] items=["[Data] Update Data", "[Scale] Update Polar Scale", "[Scale] Autoscale", "[Legend] Update Legend", "[Cursor] Cursor Release", "[Pane] Change Minimum Size", "[Annt] Upodate Annotation", "[Plot] Appearance", "[Cursor] Visibility", "[Cursor] Appearance", "[Cursor] Index", "[Scale] MagnitudeVisibility", "[Scale] PhaseVisibility", "[Scale] PhaseAppearance", "[Scale] MagnitudeApperance", "[Plot] AcceptanceRegion", "[Scale] RangeChange", "[Marker] Appearance", "[Marker] List", "[Marker] Visibility", "[Legend] Visibility", "[Legend] Color", "[Data] Index", "[Legend] Update String", "[Cursor] Trigger Event", "[Scale] Trigger Event", "[Data] Clear Graph"] ("To Do")
            w396 = bool[] []
            n215 = event-data() -> ("CtlRef"=w389:refnum<vi>, "OldVal"=w391:T10, "NewVal"=w390:T10)  [unwired: 1 in]
            n216 = Variant To Data(type=w396, Variant=w390) -> (data=w395:bool[])  [unwired: 1 in, 1 out]
            n217 = Variant To Data(type=w396, Variant=w391) -> (data=w394:bool[])  [unwired: 1 in, 1 out]
            n218 = Exclusive Or(1:w395, 2:w394) -> (0:w393:bool[])
            n219 = Search 1D Array(1D array=w393, element=TRUE) -> (index of element=w386:i32)  [unwired: 1 in]
            n220 = call <vilib>:"svx_Polar_Manage_Cluster.vi"("index"=w386, "Clust Refnum"=w389) -> ()  [unwired: 10 in]
            n221 = Bundle By Name(cluster=w387, "Plot.Line Style"=w386) -> (w385:T4)
          }
          event "Plot.Line Width": Value Change {
            w397 = T15[] [enum."[Plot] Appearance"] items=["[Data] Update Data", "[Scale] Update Polar Scale", "[Scale] Autoscale", "[Legend] Update Legend", "[Cursor] Cursor Release", "[Pane] Change Minimum Size", "[Annt] Upodate Annotation", "[Plot] Appearance", "[Cursor] Visibility", "[Cursor] Appearance", "[Cursor] Index", "[Scale] MagnitudeVisibility", "[Scale] PhaseVisibility", "[Scale] PhaseAppearance", "[Scale] MagnitudeApperance", "[Plot] AcceptanceRegion", "[Scale] RangeChange", "[Marker] Appearance", "[Marker] List", "[Marker] Visibility", "[Legend] Visibility", "[Legend] Color", "[Data] Index", "[Legend] Update String", "[Cursor] Trigger Event", "[Scale] Trigger Event", "[Data] Clear Graph"] ("To Do")
            w409 = bool[] []
            n222 = event-data() -> ("CtlRef"=w399:refnum<vi>, "OldVal"=w400:T11, "NewVal"=w401:T11)  [unwired: 1 in]
            n223 = Variant To Data(type=w409, Variant=w401) -> (data=w408:bool[])  [unwired: 1 in, 1 out]
            n224 = Variant To Data(type=w409, Variant=w400) -> (data=w407:bool[])  [unwired: 1 in, 1 out]
            n225 = Exclusive Or(1:w408, 2:w407) -> (0:w406:bool[])
            n226 = Search 1D Array(1D array=w406, element=TRUE) -> (index of element=w398:i32)  [unwired: 1 in]
            n227 = Bundle By Name(cluster=w403, "Plot.Line Width"=w398) -> (w402:T4)
            n228 = call <vilib>:"svx_Polar_Manage_Cluster.vi"("index"=w398, "Clust Refnum"=w399) -> ()  [unwired: 10 in]
          }
          event "Plot.Point Style": Value Change {
            w410 = T15[] [enum."[Plot] Appearance"] items=["[Data] Update Data", "[Scale] Update Polar Scale", "[Scale] Autoscale", "[Legend] Update Legend", "[Cursor] Cursor Release", "[Pane] Change Minimum Size", "[Annt] Upodate Annotation", "[Plot] Appearance", "[Cursor] Visibility", "[Cursor] Appearance", "[Cursor] Index", "[Scale] MagnitudeVisibility", "[Scale] PhaseVisibility", "[Scale] PhaseAppearance", "[Scale] MagnitudeApperance", "[Plot] AcceptanceRegion", "[Scale] RangeChange", "[Marker] Appearance", "[Marker] List", "[Marker] Visibility", "[Legend] Visibility", "[Legend] Color", "[Data] Index", "[Legend] Update String", "[Cursor] Trigger Event", "[Scale] Trigger Event", "[Data] Clear Graph"] ("To Do")
            w422 = bool[] []
            n229 = event-data() -> ("CtlRef"=w414:refnum<vi>, "OldVal"=w412:T9, "NewVal"=w413:T9)  [unwired: 1 in]
            n230 = Variant To Data(type=w422, Variant=w413) -> (data=w421:bool[])  [unwired: 1 in, 1 out]
            n231 = Variant To Data(type=w422, Variant=w412) -> (data=w420:bool[])  [unwired: 1 in, 1 out]
            n232 = Exclusive Or(1:w421, 2:w420) -> (0:w419:bool[])
            n233 = Search 1D Array(1D array=w419, element=TRUE) -> (index of element=w411:i32)  [unwired: 1 in]
            n234 = call <vilib>:"svx_Polar_Manage_Cluster.vi"("index"=w411, "Clust Refnum"=w414) -> ()  [unwired: 10 in]
            n235 = Bundle By Name(cluster=w416, "Plot.Point Style"=w411) -> (w415:T4)
          }
          event "Cursor.Line Style": Value Change {
            w423 = T15[] [enum."[Cursor] Appearance"] items=["[Data] Update Data", "[Scale] Update Polar Scale", "[Scale] Autoscale", "[Legend] Update Legend", "[Cursor] Cursor Release", "[Pane] Change Minimum Size", "[Annt] Upodate Annotation", "[Plot] Appearance", "[Cursor] Visibility", "[Cursor] Appearance", "[Cursor] Index", "[Scale] MagnitudeVisibility", "[Scale] PhaseVisibility", "[Scale] PhaseAppearance", "[Scale] MagnitudeApperance", "[Plot] AcceptanceRegion", "[Scale] RangeChange", "[Marker] Appearance", "[Marker] List", "[Marker] Visibility", "[Legend] Visibility", "[Legend] Color", "[Data] Index", "[Legend] Update String", "[Cursor] Trigger Event", "[Scale] Trigger Event", "[Data] Clear Graph"] ("To Do")
            w435 = bool[] []
            n236 = event-data() -> ("CtlRef"=w425:refnum<vi>, "OldVal"=w424:T10, "NewVal"=w426:T10)  [unwired: 1 in]
            n237 = Variant To Data(type=w435, Variant=w426) -> (data=w434:bool[])  [unwired: 1 in, 1 out]
            n238 = Variant To Data(type=w435, Variant=w424) -> (data=w433:bool[])  [unwired: 1 in, 1 out]
            n239 = Exclusive Or(1:w434, 2:w433) -> (0:w432:bool[])
            n240 = Search 1D Array(1D array=w432, element=TRUE) -> (index of element=w427:i32)  [unwired: 1 in]
            n241 = call <vilib>:"svx_Polar_Manage_Cluster.vi"("index"=w427, "Clust Refnum"=w425) -> ()  [unwired: 10 in]
            n242 = Bundle By Name(cluster=w429, "Cursor.Line Style"=w427) -> (w428:T4)
          }
          event "Cursor.Line Width": Value Change {
            w436 = T15[] [enum."[Cursor] Appearance"] items=["[Data] Update Data", "[Scale] Update Polar Scale", "[Scale] Autoscale", "[Legend] Update Legend", "[Cursor] Cursor Release", "[Pane] Change Minimum Size", "[Annt] Upodate Annotation", "[Plot] Appearance", "[Cursor] Visibility", "[Cursor] Appearance", "[Cursor] Index", "[Scale] MagnitudeVisibility", "[Scale] PhaseVisibility", "[Scale] PhaseAppearance", "[Scale] MagnitudeApperance", "[Plot] AcceptanceRegion", "[Scale] RangeChange", "[Marker] Appearance", "[Marker] List", "[Marker] Visibility", "[Legend] Visibility", "[Legend] Color", "[Data] Index", "[Legend] Update String", "[Cursor] Trigger Event", "[Scale] Trigger Event", "[Data] Clear Graph"] ("To Do")
            w448 = bool[] []
            n243 = event-data() -> ("CtlRef"=w439:refnum<vi>, "OldVal"=w438:T11, "NewVal"=w437:T11)  [unwired: 1 in]
            n244 = Variant To Data(type=w448, Variant=w437) -> (data=w447:bool[])  [unwired: 1 in, 1 out]
            n245 = Variant To Data(type=w448, Variant=w438) -> (data=w446:bool[])  [unwired: 1 in, 1 out]
            n246 = Exclusive Or(1:w447, 2:w446) -> (0:w445:bool[])
            n247 = Search 1D Array(1D array=w445, element=TRUE) -> (index of element=w440:i32)  [unwired: 1 in]
            n248 = call <vilib>:"svx_Polar_Manage_Cluster.vi"("index"=w440, "Clust Refnum"=w439) -> ()  [unwired: 10 in]
            n249 = Bundle By Name(cluster=w442, "Cursor.Line Width"=w440) -> (w441:T4)
          }
          event "Cursor.Point Style": Value Change {
            w449 = T15[] [enum."[Cursor] Appearance"] items=["[Data] Update Data", "[Scale] Update Polar Scale", "[Scale] Autoscale", "[Legend] Update Legend", "[Cursor] Cursor Release", "[Pane] Change Minimum Size", "[Annt] Upodate Annotation", "[Plot] Appearance", "[Cursor] Visibility", "[Cursor] Appearance", "[Cursor] Index", "[Scale] MagnitudeVisibility", "[Scale] PhaseVisibility", "[Scale] PhaseAppearance", "[Scale] MagnitudeApperance", "[Plot] AcceptanceRegion", "[Scale] RangeChange", "[Marker] Appearance", "[Marker] List", "[Marker] Visibility", "[Legend] Visibility", "[Legend] Color", "[Data] Index", "[Legend] Update String", "[Cursor] Trigger Event", "[Scale] Trigger Event", "[Data] Clear Graph"] ("To Do")
            w461 = bool[] []
            n250 = event-data() -> ("CtlRef"=w452:refnum<vi>, "OldVal"=w451:T9, "NewVal"=w450:T9)  [unwired: 1 in]
            n251 = Variant To Data(type=w461, Variant=w450) -> (data=w460:bool[])  [unwired: 1 in, 1 out]
            n252 = Variant To Data(type=w461, Variant=w451) -> (data=w459:bool[])  [unwired: 1 in, 1 out]
            n253 = Exclusive Or(1:w460, 2:w459) -> (0:w458:bool[])
            n254 = Search 1D Array(1D array=w458, element=TRUE) -> (index of element=w453:i32)  [unwired: 1 in]
            n255 = Bundle By Name(cluster=w455, "Cursor.Point Style"=w453) -> (w454:T4)
            n256 = call <vilib>:"svx_Polar_Manage_Cluster.vi"("index"=w453, "Clust Refnum"=w452) -> ()  [unwired: 10 in]
          }
          event "Cursor.Style": Value Change {
            w462 = T15[] [enum."[Cursor] Appearance"] items=["[Data] Update Data", "[Scale] Update Polar Scale", "[Scale] Autoscale", "[Legend] Update Legend", "[Cursor] Cursor Release", "[Pane] Change Minimum Size", "[Annt] Upodate Annotation", "[Plot] Appearance", "[Cursor] Visibility", "[Cursor] Appearance", "[Cursor] Index", "[Scale] MagnitudeVisibility", "[Scale] PhaseVisibility", "[Scale] PhaseAppearance", "[Scale] MagnitudeApperance", "[Plot] AcceptanceRegion", "[Scale] RangeChange", "[Marker] Appearance", "[Marker] List", "[Marker] Visibility", "[Legend] Visibility", "[Legend] Color", "[Data] Index", "[Legend] Update String", "[Cursor] Trigger Event", "[Scale] Trigger Event", "[Data] Clear Graph"] ("To Do")
            w474 = bool[] []
            n257 = event-data() -> ("CtlRef"=w465:refnum<vi>, "OldVal"=w464:T12, "NewVal"=w463:T12)  [unwired: 1 in]
            n258 = Variant To Data(type=w474, Variant=w463) -> (data=w473:bool[])  [unwired: 1 in, 1 out]
            n259 = Variant To Data(type=w474, Variant=w464) -> (data=w472:bool[])  [unwired: 1 in, 1 out]
            n260 = Exclusive Or(1:w473, 2:w472) -> (0:w471:bool[])
            n261 = Search 1D Array(1D array=w471, element=TRUE) -> (index of element=w466:i32)  [unwired: 1 in]
            n262 = call <vilib>:"svx_Polar_Manage_Cluster.vi"("index"=w466, "Clust Refnum"=w465) -> ()  [unwired: 10 in]
            n263 = Bundle By Name(cluster=w468, "Cursor.Style"=w466) -> (w467:T4)
          }
          event "Marker.Point Style": Value Change {
            w475 = T15[] [enum."[Marker] Appearance"] items=["[Data] Update Data", "[Scale] Update Polar Scale", "[Scale] Autoscale", "[Legend] Update Legend", "[Cursor] Cursor Release", "[Pane] Change Minimum Size", "[Annt] Upodate Annotation", "[Plot] Appearance", "[Cursor] Visibility", "[Cursor] Appearance", "[Cursor] Index", "[Scale] MagnitudeVisibility", "[Scale] PhaseVisibility", "[Scale] PhaseAppearance", "[Scale] MagnitudeApperance", "[Plot] AcceptanceRegion", "[Scale] RangeChange", "[Marker] Appearance", "[Marker] List", "[Marker] Visibility", "[Legend] Visibility", "[Legend] Color", "[Data] Index", "[Legend] Update String", "[Cursor] Trigger Event", "[Scale] Trigger Event", "[Data] Clear Graph"] ("To Do")
            w487 = bool[] []
            n264 = event-data() -> ("CtlRef"=w478:refnum<vi>, "OldVal"=w477:T9, "NewVal"=w476:T9)  [unwired: 1 in]
            n265 = Variant To Data(type=w487, Variant=w476) -> (data=w486:bool[])  [unwired: 1 in, 1 out]
            n266 = Variant To Data(type=w487, Variant=w477) -> (data=w485:bool[])  [unwired: 1 in, 1 out]
            n267 = Exclusive Or(1:w486, 2:w485) -> (0:w484:bool[])
            n268 = Search 1D Array(1D array=w484, element=TRUE) -> (index of element=w479:i32)  [unwired: 1 in]
            n269 = Bundle By Name(cluster=w480, "Marker.Point Style"=w479) -> (w481:T4)
            n270 = call <vilib>:"svx_Polar_Manage_Cluster.vi"("index"=w479, "Clust Refnum"=w478) -> ()  [unwired: 10 in]
          }
          event "Marker.Style": Value Change {
            w488 = T15[] [enum."[Marker] Appearance"] items=["[Data] Update Data", "[Scale] Update Polar Scale", "[Scale] Autoscale", "[Legend] Update Legend", "[Cursor] Cursor Release", "[Pane] Change Minimum Size", "[Annt] Upodate Annotation", "[Plot] Appearance", "[Cursor] Visibility", "[Cursor] Appearance", "[Cursor] Index", "[Scale] MagnitudeVisibility", "[Scale] PhaseVisibility", "[Scale] PhaseAppearance", "[Scale] MagnitudeApperance", "[Plot] AcceptanceRegion", "[Scale] RangeChange", "[Marker] Appearance", "[Marker] List", "[Marker] Visibility", "[Legend] Visibility", "[Legend] Color", "[Data] Index", "[Legend] Update String", "[Cursor] Trigger Event", "[Scale] Trigger Event", "[Data] Clear Graph"] ("To Do")
            w500 = bool[] []
            n271 = event-data() -> ("CtlRef"=w491:refnum<vi>, "OldVal"=w489:T12, "NewVal"=w490:T12)  [unwired: 1 in]
            n272 = Variant To Data(type=w500, Variant=w490) -> (data=w499:bool[])  [unwired: 1 in, 1 out]
            n273 = Variant To Data(type=w500, Variant=w489) -> (data=w498:bool[])  [unwired: 1 in, 1 out]
            n274 = Exclusive Or(1:w499, 2:w498) -> (0:w497:bool[])
            n275 = Search 1D Array(1D array=w497, element=TRUE) -> (index of element=w492:i32)  [unwired: 1 in]
            n276 = call <vilib>:"svx_Polar_Manage_Cluster.vi"("index"=w492, "Clust Refnum"=w491) -> ()  [unwired: 10 in]
            n277 = Bundle By Name(cluster=w493, "Marker.Style"=w492) -> (w494:T4)
          }
          event "Marker.Visible": Value Change {
            w501 = T15[] [enum."[Marker] Visibility"] items=["[Data] Update Data", "[Scale] Update Polar Scale", "[Scale] Autoscale", "[Legend] Update Legend", "[Cursor] Cursor Release", "[Pane] Change Minimum Size", "[Annt] Upodate Annotation", "[Plot] Appearance", "[Cursor] Visibility", "[Cursor] Appearance", "[Cursor] Index", "[Scale] MagnitudeVisibility", "[Scale] PhaseVisibility", "[Scale] PhaseAppearance", "[Scale] MagnitudeApperance", "[Plot] AcceptanceRegion", "[Scale] RangeChange", "[Marker] Appearance", "[Marker] List", "[Marker] Visibility", "[Legend] Visibility", "[Legend] Color", "[Data] Index", "[Legend] Update String", "[Cursor] Trigger Event", "[Scale] Trigger Event", "[Data] Clear Graph"] ("To Do")
            n278 = event-data() -> ("NewVal"=w503:bool)  [unwired: 1 in]
            n279 = Bundle By Name(cluster=w504, "Marker:Visible"=w503) -> (w502:T4)
          }
          event "AR.Add": Value Change {
            w506 = T15[] [enum."[Plot] AcceptanceRegion"] items=["[Data] Update Data", "[Scale] Update Polar Scale", "[Scale] Autoscale", "[Legend] Update Legend", "[Cursor] Cursor Release", "[Pane] Change Minimum Size", "[Annt] Upodate Annotation", "[Plot] Appearance", "[Cursor] Visibility", "[Cursor] Appearance", "[Cursor] Index", "[Scale] MagnitudeVisibility", "[Scale] PhaseVisibility", "[Scale] PhaseAppearance", "[Scale] MagnitudeApperance", "[Plot] AcceptanceRegion", "[Scale] RangeChange", "[Marker] Appearance", "[Marker] List", "[Marker] Visibility", "[Legend] Visibility", "[Legend] Color", "[Data] Index", "[Legend] Update String", "[Cursor] Trigger Event", "[Scale] Trigger Event", "[Data] Clear Graph"] ("To Do")
            w509 = u8 0 ("Disabled")
            n280 = event-data() -> ()  [unwired: 1 in, 1 out]
            n281 = property on="AR.Name" class="Str"("Disabled"=w509) -> ()  [unwired: 2 in, 2 out]
            n282 = Unbundle By Name(w534) -> ("Indication Arcs"=w536:T5)
            n283 = Index Array(array=T5 [{"Name"="", "Start radius"=0.0, "End radius"=0.0, "Line Style"=0, "Line Width"=0, "Border color"=0, "Fill color"=16777216, "Start angle"=0, "End angle"=360, "Visible"=TRUE}] ("Indication Arcs")) -> (element=w511:T14)  [unwired: 1 in]
            n284 = property on="AR.Visible" class="Bool (strict)"("Disabled"=w509) -> ()  [unwired: 2 in, 2 out]
            n285 = Array Size(array=w536) -> (size(s)=w513:i32)
            n286 = Unbundle By Name(w511) -> ("Start radius"=w512:dbl, "End radius"=w529:dbl, "Line Style"=w528:i32, "Line Width"=w527:i32, "Border color"=w526:u32, "Start angle"=w525:i16, "End angle"=w524:i16, "Visible"=w523:bool, "Fill color"=w508:u32)
            n287 = property on="AR.Selector" class="Ring (strict)"("Disabled"=w509) -> ()  [unwired: 2 in, 2 out]
            n288 = Number To Decimal String(number=w513) -> (decimal integer string=w537:string)  [unwired: 1 in]
            n289 = Concatenate Strings("Acceptance Region " ("string"), w537) -> (w518:string)
            n290 = local write "AR.End Radius"(w529) -> ()
            n291 = local write "AR.End Angle"(w524) -> ()
            n292 = local write "AR.Fill Color"(w508) -> ()
            n293 = property on="AR.Start Angle" class="DigNum (strict)"("Disabled"=w509) -> ()  [unwired: 2 in, 2 out]
            n294 = local write "AR.Color"(w526) -> ()
            n295 = Bundle By Name(cluster=w511, "Name"=w518) -> (w535:T14)
            n296 = local write "AR.Start Radius"(w512) -> ()
            n297 = property on="AR.Width" class="Clust (strict)"("Disabled"=w509) -> ()  [unwired: 2 in, 2 out]
            n298 = local write "AR.Start Angle"(w525) -> ()
            n299 = local write "AR.Visible"(w523) -> ()
            n300 = Build Array (concatenate)(w536, w535) -> (w533:T5)
            n301 = property on="AR.Selector" class="Ring (strict)"() -> ("Strings []"=w520:string[])  [unwired: 2 in, 2 out]
            n302 = property on="AR.Style" class="Clust (strict)"("Disabled"=w509) -> ()  [unwired: 2 in, 2 out]
            n303 = local write "AR.Name"(w518) -> ()
            n304 = control-ref of="AR.Style"() -> (w531:refnum<vi>)
            n305 = control-ref of="AR.Width"() -> (w530:refnum<vi>)
            n306 = Build Array (concatenate)(w520, w518) -> (w516:string[])
            n307 = Build Array(w518) -> (w517:string[])
            n308 = property on="AR.Start Radius" class="DigNum (strict)"("Disabled"=w509) -> ()  [unwired: 2 in, 2 out]
            n309 = Bundle By Name(cluster=w534, "Indication Arcs"=w533, "Arc.Selector"=w513) -> (w521:T4)
            n310 = Equal To 0?(x=w513) -> (x = 0?=w519:bool)
            n311 = call <vilib>:"svx_Polar_Manage_Cluster.vi"("index"=w528, "Clust Refnum"=w531) -> ()  [unwired: 10 in]
            n312 = call <vilib>:"svx_Polar_Manage_Cluster.vi"("index"=w527, "Clust Refnum"=w530) -> ()  [unwired: 10 in]
            n313 = property on="AR.End Radius" class="DigNum (strict)"("Disabled"=w509) -> ()  [unwired: 2 in, 2 out]
            n314 = Select(t=w517, s=w519, f=w516) -> (s? t:f=w515:string[])
            n315 = property on="AR.End Angle" class="DigNum (strict)"("Disabled"=w509) -> ()  [unwired: 2 in, 2 out]
            n316 = local write "AR.Selector"(w513) -> ()
            n317 = property on="AR.Selector" class="Ring (strict)"("Strings []"=w515, "Disabled Items []"=i32[] []) -> ()  [unwired: 2 in, 2 out]
            n318 = property on="AR.Color" class="ColBox"("Disabled"=w509) -> (error out=w510:errorcluster)  [unwired: 2 in, 1 out]
            n319 = property on="AR.Fill Color" class="ColBox"(error in=w510, "Disabled"=w509) -> ()  [unwired: 1 in, 2 out]
          }
          event "AR.Remove": Value Change {
            w538 = T15[] [enum."[Plot] AcceptanceRegion"] items=["[Data] Update Data", "[Scale] Update Polar Scale", "[Scale] Autoscale", "[Legend] Update Legend", "[Cursor] Cursor Release", "[Pane] Change Minimum Size", "[Annt] Upodate Annotation", "[Plot] Appearance", "[Cursor] Visibility", "[Cursor] Appearance", "[Cursor] Index", "[Scale] MagnitudeVisibility", "[Scale] PhaseVisibility", "[Scale] PhaseAppearance", "[Scale] MagnitudeApperance", "[Plot] AcceptanceRegion", "[Scale] RangeChange", "[Marker] Appearance", "[Marker] List", "[Marker] Visibility", "[Legend] Visibility", "[Legend] Color", "[Data] Index", "[Legend] Update String", "[Cursor] Trigger Event", "[Scale] Trigger Event", "[Data] Clear Graph"] ("To Do")
            n320 = event-data() -> ()  [unwired: 1 in, 1 out]
            n321 = Unbundle By Name(w572) -> ("Indication Arcs"=w559:T5)
            n322 = local read "AR.Selector"() -> (w557:u16)
            n323 = property on="AR.Selector" class="Ring (strict)"() -> ("Strings []"=w558:string[])  [unwired: 2 in, 2 out]
            n324 = Delete From Array(array=w559, index=w557) -> (array with subset deleted=w552:T5)  [unwired: 1 in, 1 out]
            n325 = Delete From Array(array=w558, index=w557) -> (array with subset deleted=w549:string[])  [unwired: 1 in, 1 out]
            n326 = Array Size(array=w552) -> (size(s)=w551:i32)
            n327 = To Word Integer(number=w557) -> (16bit integer=w556:i16)
            n328 = Equal To 0?(x=w551) -> (x = 0?=w546:bool)
            n329 = Boolean To (0,1)(Boolean=w546) -> (0, 1=w550:i16)
            n330 = Select(t=string[] ["Acceptance Region 0"], s=w546, f=w549) -> (s? t:f=w547:string[])
            n331 = Select(t=i32[] [1] ("Disabled Items []"), s=w546, f=i32[] [] ("Disabled Items []")) -> (s? t:f=w543:i32[])
            n332 = Add(x=w550, y=w550) -> (x+y=w540:i16)
            n333 = property on="AR.Name" class="Str"("Disabled"=w540) -> ()  [unwired: 2 in, 2 out]
            n334 = property on="AR.Visible" class="Bool (strict)"("Disabled"=w540) -> ()  [unwired: 2 in, 2 out]
            n335 = property on="AR.Selector" class="Ring (strict)"("Disabled"=w540) -> ()  [unwired: 2 in, 2 out]
            n336 = property on="AR.Start Angle" class="DigNum (strict)"("Disabled"=w540) -> ()  [unwired: 2 in, 2 out]
            n337 = property on="AR.Width" class="Clust (strict)"("Disabled"=w540) -> ()  [unwired: 2 in, 2 out]
            n338 = Decrement(x=w556) -> (x-1=w555:i16)
            n339 = property on="AR.Style" class="Clust (strict)"("Disabled"=w540) -> ()  [unwired: 2 in, 2 out]
            n340 = Max & Min(x=w555, y=i16 0) -> (max(x,y)=w542:i16)  [unwired: 1 out]
            n341 = property on="AR.Start Radius" class="DigNum (strict)"("Disabled"=w540) -> ()  [unwired: 2 in, 2 out]
            n342 = Index Array(array=w552, index=w542) -> (element=w553:T14)
            n343 = Unbundle By Name(w553) -> ("Name"=w560:string, "Start radius"=w569:dbl, "End radius"=w541:dbl, "Line Style"=w568:i32, "Line Width"=w567:i32, "Border color"=w566:u32, "Start angle"=w565:i16, "End angle"=w564:i16, "Visible"=w563:bool, "Fill color"=w539:u32)
            n344 = local write "AR.Start Radius"(w569) -> ()
            n345 = local write "AR.End Angle"(w564) -> ()
            n346 = local write "AR.Fill Color"(w539) -> ()
            n347 = local write "AR.Color"(w566) -> ()
            n348 = local write "AR.End Radius"(w541) -> ()
            n349 = local write "AR.Start Angle"(w565) -> ()
            n350 = Bundle By Name(cluster=w572, "Indication Arcs"=w552, "Arc.Selector"=w542) -> (w561:T4)
            n351 = local write "AR.Name"(w560) -> ()
            n352 = local write "AR.Visible"(w563) -> ()
            n353 = property on="AR.End Radius" class="DigNum (strict)"("Disabled"=w540) -> ()  [unwired: 2 in, 2 out]
            n354 = local write "AR.Selector"(w542) -> ()
            n355 = control-ref of="AR.Style"() -> (w571:refnum<vi>)
            n356 = control-ref of="AR.Width"() -> (w570:refnum<vi>)
            n357 = property on="AR.End Angle" class="DigNum (strict)"("Disabled"=w540) -> ()  [unwired: 2 in, 2 out]
            n358 = property on="AR.Selector" class="Ring (strict)"("Strings []"=w547, "Disabled Items []"=w543) -> ()  [unwired: 2 in, 2 out]
            n359 = property on="AR.Color" class="ColBox"("Disabled"=w540) -> ()  [unwired: 2 in, 2 out]
            n360 = property on="AR.Fill Color" class="ColBox"("Disabled"=w540) -> ()  [unwired: 2 in, 2 out]
            n361 = call <vilib>:"svx_Polar_Manage_Cluster.vi"("index"=w568, "Clust Refnum"=w571) -> ()  [unwired: 10 in]
            n362 = call <vilib>:"svx_Polar_Manage_Cluster.vi"("index"=w567, "Clust Refnum"=w570) -> ()  [unwired: 10 in]
          }
          event "AR.Selector": Value Change {
            n363 = event-data() -> ("NewVal"=w587:u16)  [unwired: 1 in]
            n364 = Unbundle By Name(w589) -> ("Indication Arcs"=w588:T5)
            n365 = Index Array(array=w588, index=w587) -> (element=w586:T14)
            n366 = Unbundle By Name(w586) -> ("Name"=w583:string, "Start radius"=w582:dbl, "End radius"=w574:dbl, "Line Style"=w581:i32, "Line Width"=w580:i32, "Border color"=w579:u32, "Start angle"=w578:i16, "End angle"=w577:i16, "Visible"=w576:bool, "Fill color"=w573:u32)
            n367 = local write "AR.Start Radius"(w582) -> ()
            n368 = local write "AR.End Angle"(w577) -> ()
            n369 = local write "AR.Fill Color"(w573) -> ()
            n370 = local write "AR.Color"(w579) -> ()
            n371 = local write "AR.End Radius"(w574) -> ()
            n372 = local write "AR.Start Angle"(w578) -> ()
            n373 = local write "AR.Name"(w583) -> ()
            n374 = local write "AR.Visible"(w576) -> ()
            n375 = control-ref of="AR.Style"() -> (w585:refnum<vi>)
            n376 = control-ref of="AR.Width"() -> (w584:refnum<vi>)
            n377 = call <vilib>:"svx_Polar_Manage_Cluster.vi"("index"=w581, "Clust Refnum"=w585) -> ()  [unwired: 10 in]
            n378 = call <vilib>:"svx_Polar_Manage_Cluster.vi"("index"=w580, "Clust Refnum"=w584) -> ()  [unwired: 10 in]
          }
          event "AR.Start Radius": Value Change {
            w590 = T15[] [enum."[Plot] AcceptanceRegion"] items=["[Data] Update Data", "[Scale] Update Polar Scale", "[Scale] Autoscale", "[Legend] Update Legend", "[Cursor] Cursor Release", "[Pane] Change Minimum Size", "[Annt] Upodate Annotation", "[Plot] Appearance", "[Cursor] Visibility", "[Cursor] Appearance", "[Cursor] Index", "[Scale] MagnitudeVisibility", "[Scale] PhaseVisibility", "[Scale] PhaseAppearance", "[Scale] MagnitudeApperance", "[Plot] AcceptanceRegion", "[Scale] RangeChange", "[Marker] Appearance", "[Marker] List", "[Marker] Visibility", "[Legend] Visibility", "[Legend] Color", "[Data] Index", "[Legend] Update String", "[Cursor] Trigger Event", "[Scale] Trigger Event", "[Data] Clear Graph"] ("To Do")
            n379 = event-data() -> ("NewVal"=w592:dbl)  [unwired: 1 in]
            n380 = Unbundle By Name(w600) -> ("Indication Arcs"=w603:T5)
            n381 = local read "AR.Selector"() -> (w601:u16)
            n382 = Index Array(array=w603, index=w601) -> (element=w596:T14)
            n383 = Unbundle By Name(w596) -> ("Start radius"=w595:dbl, "End radius"=w593:dbl)
            n384 = Equal?(x=w595, y=w593) -> (x = y?=w594:bool)
            n385 = Select(t=w592, s=w594, f=w593) -> (s? t:f=w591:dbl)
            n386 = Bundle By Name(cluster=w596, "Start radius"=w592, "End radius"=w591) -> (w602:T14)
            n387 = local write "AR.End Radius"(w591) -> ()
            n388 = Replace Array Subset(array=w603, new element=w602, index=w601) -> (w599:T5)
            n389 = Bundle By Name(cluster=w600, "Indication Arcs"=w599) -> (w597:T4)
          }
          event "AR.End Radius": Value Change {
            w604 = T15[] [enum."[Plot] AcceptanceRegion"] items=["[Data] Update Data", "[Scale] Update Polar Scale", "[Scale] Autoscale", "[Legend] Update Legend", "[Cursor] Cursor Release", "[Pane] Change Minimum Size", "[Annt] Upodate Annotation", "[Plot] Appearance", "[Cursor] Visibility", "[Cursor] Appearance", "[Cursor] Index", "[Scale] MagnitudeVisibility", "[Scale] PhaseVisibility", "[Scale] PhaseAppearance", "[Scale] MagnitudeApperance", "[Plot] AcceptanceRegion", "[Scale] RangeChange", "[Marker] Appearance", "[Marker] List", "[Marker] Visibility", "[Legend] Visibility", "[Legend] Color", "[Data] Index", "[Legend] Update String", "[Cursor] Trigger Event", "[Scale] Trigger Event", "[Data] Clear Graph"] ("To Do")
            n390 = event-data() -> ("NewVal"=w605:dbl)  [unwired: 1 in]
            n391 = Unbundle By Name(w610) -> ("Indication Arcs"=w613:T5)
            n392 = local read "AR.Selector"() -> (w611:u16)
            n393 = Index Array(array=w613, index=w611) -> (element=w606:T14)
            n394 = Bundle By Name(cluster=w606, "End radius"=w605) -> (w612:T14)
            n395 = Replace Array Subset(array=w613, new element=w612, index=w611) -> (w609:T5)
            n396 = Bundle By Name(cluster=w610, "Indication Arcs"=w609) -> (w607:T4)
          }
          event "AR.Start Angle": Value Change {
            w614 = T15[] [enum."[Plot] AcceptanceRegion"] items=["[Data] Update Data", "[Scale] Update Polar Scale", "[Scale] Autoscale", "[Legend] Update Legend", "[Cursor] Cursor Release", "[Pane] Change Minimum Size", "[Annt] Upodate Annotation", "[Plot] Appearance", "[Cursor] Visibility", "[Cursor] Appearance", "[Cursor] Index", "[Scale] MagnitudeVisibility", "[Scale] PhaseVisibility", "[Scale] PhaseAppearance", "[Scale] MagnitudeApperance", "[Plot] AcceptanceRegion", "[Scale] RangeChange", "[Marker] Appearance", "[Marker] List", "[Marker] Visibility", "[Legend] Visibility", "[Legend] Color", "[Data] Index", "[Legend] Update String", "[Cursor] Trigger Event", "[Scale] Trigger Event", "[Data] Clear Graph"] ("To Do")
            n397 = event-data() -> ("NewVal"=w622:i16)  [unwired: 1 in]
            n398 = Unbundle By Name(w618) -> ("Indication Arcs"=w621:T5)
            n399 = local read "AR.Selector"() -> (w619:u16)
            n400 = Index Array(array=w621, index=w619) -> (element=w623:T14)
            n401 = Bundle By Name(cluster=w623, "Start angle"=w622) -> (w620:T14)
            n402 = Replace Array Subset(array=w621, new element=w620, index=w619) -> (w617:T5)
            n403 = Bundle By Name(cluster=w618, "Indication Arcs"=w617) -> (w615:T4)
          }
          event "AR.End Angle": Value Change {
            w624 = T15[] [enum."[Plot] AcceptanceRegion"] items=["[Data] Update Data", "[Scale] Update Polar Scale", "[Scale] Autoscale", "[Legend] Update Legend", "[Cursor] Cursor Release", "[Pane] Change Minimum Size", "[Annt] Upodate Annotation", "[Plot] Appearance", "[Cursor] Visibility", "[Cursor] Appearance", "[Cursor] Index", "[Scale] MagnitudeVisibility", "[Scale] PhaseVisibility", "[Scale] PhaseAppearance", "[Scale] MagnitudeApperance", "[Plot] AcceptanceRegion", "[Scale] RangeChange", "[Marker] Appearance", "[Marker] List", "[Marker] Visibility", "[Legend] Visibility", "[Legend] Color", "[Data] Index", "[Legend] Update String", "[Cursor] Trigger Event", "[Scale] Trigger Event", "[Data] Clear Graph"] ("To Do")
            n404 = event-data() -> ("NewVal"=w632:i16)  [unwired: 1 in]
            n405 = Unbundle By Name(w628) -> ("Indication Arcs"=w631:T5)
            n406 = local read "AR.Selector"() -> (w629:u16)
            n407 = Index Array(array=w631, index=w629) -> (element=w633:T14)
            n408 = Bundle By Name(cluster=w633, "End angle"=w632) -> (w630:T14)
            n409 = Replace Array Subset(array=w631, new element=w630, index=w629) -> (w627:T5)
            n410 = Bundle By Name(cluster=w628, "Indication Arcs"=w627) -> (w625:T4)
          }
          event "AR.Color": Value Change {
            w634 = T15[] [enum."[Plot] AcceptanceRegion"] items=["[Data] Update Data", "[Scale] Update Polar Scale", "[Scale] Autoscale", "[Legend] Update Legend", "[Cursor] Cursor Release", "[Pane] Change Minimum Size", "[Annt] Upodate Annotation", "[Plot] Appearance", "[Cursor] Visibility", "[Cursor] Appearance", "[Cursor] Index", "[Scale] MagnitudeVisibility", "[Scale] PhaseVisibility", "[Scale] PhaseAppearance", "[Scale] MagnitudeApperance", "[Plot] AcceptanceRegion", "[Scale] RangeChange", "[Marker] Appearance", "[Marker] List", "[Marker] Visibility", "[Legend] Visibility", "[Legend] Color", "[Data] Index", "[Legend] Update String", "[Cursor] Trigger Event", "[Scale] Trigger Event", "[Data] Clear Graph"] ("To Do")
            n411 = event-data() -> ("NewVal"=w642:u32)  [unwired: 1 in]
            n412 = Unbundle By Name(w638) -> ("Indication Arcs"=w641:T5)
            n413 = local read "AR.Selector"() -> (w639:u16)
            n414 = Index Array(array=w641, index=w639) -> (element=w643:T14)
            n415 = Bundle By Name(cluster=w643, "Border color"=w642) -> (w640:T14)
            n416 = Replace Array Subset(array=w641, new element=w640, index=w639) -> (w637:T5)
            n417 = Bundle By Name(cluster=w638, "Indication Arcs"=w637) -> (w635:T4)
          }
          event "AR.Fill Color": Value Change {
            w644 = T15[] [enum."[Plot] AcceptanceRegion"] items=["[Data] Update Data", "[Scale] Update Polar Scale", "[Scale] Autoscale", "[Legend] Update Legend", "[Cursor] Cursor Release", "[Pane] Change Minimum Size", "[Annt] Upodate Annotation", "[Plot] Appearance", "[Cursor] Visibility", "[Cursor] Appearance", "[Cursor] Index", "[Scale] MagnitudeVisibility", "[Scale] PhaseVisibility", "[Scale] PhaseAppearance", "[Scale] MagnitudeApperance", "[Plot] AcceptanceRegion", "[Scale] RangeChange", "[Marker] Appearance", "[Marker] List", "[Marker] Visibility", "[Legend] Visibility", "[Legend] Color", "[Data] Index", "[Legend] Update String", "[Cursor] Trigger Event", "[Scale] Trigger Event", "[Data] Clear Graph"] ("To Do")
            n418 = event-data() -> ("NewVal"=w652:u32)  [unwired: 1 in]
            n419 = Unbundle By Name(w648) -> ("Indication Arcs"=w651:T5)
            n420 = local read "AR.Selector"() -> (w649:u16)
            n421 = Index Array(array=w651, index=w649) -> (element=w653:T14)
            n422 = Bundle By Name(cluster=w653, "Fill color"=w652) -> (w650:T14)
            n423 = Replace Array Subset(array=w651, new element=w650, index=w649) -> (w647:T5)
            n424 = Bundle By Name(cluster=w648, "Indication Arcs"=w647) -> (w645:T4)
          }
          event "AR.Visible": Value Change {
            w654 = T15[] [enum."[Plot] AcceptanceRegion"] items=["[Data] Update Data", "[Scale] Update Polar Scale", "[Scale] Autoscale", "[Legend] Update Legend", "[Cursor] Cursor Release", "[Pane] Change Minimum Size", "[Annt] Upodate Annotation", "[Plot] Appearance", "[Cursor] Visibility", "[Cursor] Appearance", "[Cursor] Index", "[Scale] MagnitudeVisibility", "[Scale] PhaseVisibility", "[Scale] PhaseAppearance", "[Scale] MagnitudeApperance", "[Plot] AcceptanceRegion", "[Scale] RangeChange", "[Marker] Appearance", "[Marker] List", "[Marker] Visibility", "[Legend] Visibility", "[Legend] Color", "[Data] Index", "[Legend] Update String", "[Cursor] Trigger Event", "[Scale] Trigger Event", "[Data] Clear Graph"] ("To Do")
            n425 = event-data() -> ("NewVal"=w662:bool)  [unwired: 1 in]
            n426 = Unbundle By Name(w658) -> ("Indication Arcs"=w661:T5)
            n427 = local read "AR.Selector"() -> (w659:u16)
            n428 = Index Array(array=w661, index=w659) -> (element=w663:T14)
            n429 = Bundle By Name(cluster=w663, "Visible"=w662) -> (w660:T14)
            n430 = Replace Array Subset(array=w661, new element=w660, index=w659) -> (w657:T5)
            n431 = Bundle By Name(cluster=w658, "Indication Arcs"=w657) -> (w655:T4)
          }
          event "AR.Width": Value Change {
            w664 = T15[] [enum."[Plot] AcceptanceRegion"] items=["[Data] Update Data", "[Scale] Update Polar Scale", "[Scale] Autoscale", "[Legend] Update Legend", "[Cursor] Cursor Release", "[Pane] Change Minimum Size", "[Annt] Upodate Annotation", "[Plot] Appearance", "[Cursor] Visibility", "[Cursor] Appearance", "[Cursor] Index", "[Scale] MagnitudeVisibility", "[Scale] PhaseVisibility", "[Scale] PhaseAppearance", "[Scale] MagnitudeApperance", "[Plot] AcceptanceRegion", "[Scale] RangeChange", "[Marker] Appearance", "[Marker] List", "[Marker] Visibility", "[Legend] Visibility", "[Legend] Color", "[Data] Index", "[Legend] Update String", "[Cursor] Trigger Event", "[Scale] Trigger Event", "[Data] Clear Graph"] ("To Do")
            w673 = bool[] []
            n432 = event-data() -> ("CtlRef"=w668:refnum<vi>, "OldVal"=w667:T11, "NewVal"=w666:T11)  [unwired: 1 in]
            n433 = Unbundle By Name(w677) -> ("Indication Arcs"=w680:T5)
            n434 = local read "AR.Selector"() -> (w678:u16)
            n435 = Index Array(array=w680, index=w678) -> (element=w681:T14)
            n436 = Variant To Data(type=w673, Variant=w666) -> (data=w672:bool[])  [unwired: 1 in, 1 out]
            n437 = Variant To Data(type=w673, Variant=w667) -> (data=w671:bool[])  [unwired: 1 in, 1 out]
            n438 = Exclusive Or(1:w672, 2:w671) -> (0:w670:bool[])
            n439 = Search 1D Array(1D array=w670, element=TRUE) -> (index of element=w665:i32)  [unwired: 1 in]
            n440 = Bundle By Name(cluster=w681, "Line Width"=w665) -> (w679:T14)
            n441 = call <vilib>:"svx_Polar_Manage_Cluster.vi"("index"=w665, "Clust Refnum"=w668) -> ()  [unwired: 10 in]
            n442 = Replace Array Subset(array=w680, new element=w679, index=w678) -> (w676:T5)
            n443 = Bundle By Name(cluster=w677, "Indication Arcs"=w676) -> (w674:T4)
          }
          event "AR.Style": Value Change {
            w682 = T15[] [enum."[Plot] AcceptanceRegion"] items=["[Data] Update Data", "[Scale] Update Polar Scale", "[Scale] Autoscale", "[Legend] Update Legend", "[Cursor] Cursor Release", "[Pane] Change Minimum Size", "[Annt] Upodate Annotation", "[Plot] Appearance", "[Cursor] Visibility", "[Cursor] Appearance", "[Cursor] Index", "[Scale] MagnitudeVisibility", "[Scale] PhaseVisibility", "[Scale] PhaseAppearance", "[Scale] MagnitudeApperance", "[Plot] AcceptanceRegion", "[Scale] RangeChange", "[Marker] Appearance", "[Marker] List", "[Marker] Visibility", "[Legend] Visibility", "[Legend] Color", "[Data] Index", "[Legend] Update String", "[Cursor] Trigger Event", "[Scale] Trigger Event", "[Data] Clear Graph"] ("To Do")
            w691 = bool[] []
            n444 = event-data() -> ("CtlRef"=w686:refnum<vi>, "OldVal"=w685:T10, "NewVal"=w684:T10)  [unwired: 1 in]
            n445 = Unbundle By Name(w695) -> ("Indication Arcs"=w698:T5)
            n446 = local read "AR.Selector"() -> (w696:u16)
            n447 = Index Array(array=w698, index=w696) -> (element=w699:T14)
            n448 = Variant To Data(type=w691, Variant=w684) -> (data=w690:bool[])  [unwired: 1 in, 1 out]
            n449 = Variant To Data(type=w691, Variant=w685) -> (data=w689:bool[])  [unwired: 1 in, 1 out]
            n450 = Exclusive Or(1:w690, 2:w689) -> (0:w688:bool[])
            n451 = Search 1D Array(1D array=w688, element=TRUE) -> (index of element=w683:i32)  [unwired: 1 in]
            n452 = Bundle By Name(cluster=w699, "Line Style"=w683) -> (w697:T14)
            n453 = call <vilib>:"svx_Polar_Manage_Cluster.vi"("index"=w683, "Clust Refnum"=w686) -> ()  [unwired: 10 in]
            n454 = Replace Array Subset(array=w698, new element=w697, index=w696) -> (w694:T5)
            n455 = Bundle By Name(cluster=w695, "Indication Arcs"=w694) -> (w692:T4)
          }
          event "AR.Name": Value Change {
            n456 = event-data() -> ("NewVal"=w701:string)  [unwired: 1 in]
            n457 = Unbundle By Name(w707) -> ("Indication Arcs"=w709:T5)
            n458 = local read "AR.Selector"() -> (w702:u16)
            n459 = property on="AR.Selector" class="Ring (strict)"() -> ("Strings []"=w703:string[])  [unwired: 2 in, 2 out]
            n460 = Index Array(array=w709, index=w702) -> (element=w710:T14)
            n461 = Bundle By Name(cluster=w710, "Name"=w701) -> (w708:T14)
            n462 = Replace Array Subset(array=w709, new element=w708, index=w702) -> (w706:T5)
            n463 = Replace Array Subset(array=w703, new element=w701, index=w702) -> (w700:string[])
            n464 = Bundle By Name(cluster=w707, "Indication Arcs"=w706) -> (w704:T4)
            n465 = property on="AR.Selector" class="Ring (strict)"("Strings []"=w700) -> ()  [unwired: 2 in, 2 out]
          }
        }
        n466 = call <vilib>:"svx_Polar_Execute.vi"("Container State"=w159, "Polar Plot"=w167, "Plot Legend"=w166, "z scale graph"=w165, "Cursor Info"=w164, "Facade VI"=w163, "current state"=w169, "To Do"=w162, "Data In"=w161) -> ("Data Out"=w160:T1, "Display State Out"=w168:T4)  [unwired: 9 in]
      }
    }
  }
  "Action out" <- w13
  "State out" <- w16
  "Data out" <- w3
  n467 = invoke class="VI" method="FP.Close"(reference=w6) -> ()  [unwired: 2 in, 3 out]
